vi "Auto.vi"() -> ()   [LabVIEW 2017]
uses:
  Control/Saurabh/prosucer_consumer_enum.ctl
  <vilib>/addons/database/NI_Database_API.lvlib
  Global/Global 1.vi
  <vilib>/Utility/file.llb/Read Delimited Spreadsheet (string).vi
  Global/DATA LOG.vi
  <vilib>/Utility/error.llb/DialogType.ctl
  <userlib>/_OpenG.lib/comparison/comparison.llb/String Changed__ogtk.vi
  <vilib>/addons/database/Connection.llb/DB Tools Open Connec (String).vi
panel:
  out "LOG DATA":string
  out "scanner value":string
  out "PRIVIOUS DATA":string
  out "array w/ subset deleted":dbl[](array[numeric])
  out "LOG DATA 2":dbl[](array[numeric])
  out "DATA":bool
  out "Boolean 6":bool
  out "Input 3":string
  out "resulting string":string
  out "error out 5":errorcluster
  out "BARCODE RECIPE 2":string(combo)
  out "match substring":string
  out "SHIFT_DATA":string[](array[string])
  out "length 2":i32
  out "length":i32
  out "Boolean 5":bool
  out "OP40 BARCODE STRING EMPRTY":bool
  out "OP30 BARCODE STRING EMPRTY":bool
  out "trimmed string":string
  out "Array":string[][](array[string])
  out "error out 3":errorcluster
  out "OP 61":T1 {"Cycle Time" format="%#.2g"; "Actual Flow (Lpm)" format="%#.2g"; "Pressure (Bar)" format="%#.2g"; "lt Pressure (Bar)" format="%#.2g"; "Actual Flow (ccm)" format="%#.2g"}
  out "error out":errorcluster
  out "OP 10 & OP 21":T2 {"SPRING AND SEAL PRESS CHECK LOAD(N)" format="%#.2g"; "CYCLE TIME" format="%#.2g"; "SPRING AND SEAL PRESS LOAD(N)" format="%#.2g"; "SPRING LOAD AT 13.4 mm(N)" format="%#.2g"; "SPRING LOAD AT 14 mm((N)" format="%#.2g"; "SPRING HEIGHT(mm)" format="%#.2g"; "SEAL PRESS LOAD(N)" format="%#.2g"}
  out "PLC COM.":bool
  out "STATION-4 2":T3 {"PARAMETER 10" format="%#.2g"; "PARAMETER 6" format="%#.2g"; "PARAMETER 7" format="%#.2g"; "PARAMETER 9" format="%#.2g"; "PARAMETER 8" format="%#.2g"; "CYCLE TIME" format="%#.2g"; "PARAMETER 5" format="%#.2g"; "PARAMETER 1" format="%#.2g"; "PARAMETER 2" format="%#.2g"; "PARAMETER 4" format="%#.2g"; "PARAMETER 3" format="%#.2g"}
  out "STATION-3 2":T3 {"PARAMETER 10" format="%#.2g"; "PARAMETER 6" format="%#.2g"; "PARAMETER 7" format="%#.2g"; "PARAMETER 9" format="%#.2g"; "PARAMETER 8" format="%#.2g"; "CYCLE TIME" format="%#.2g"; "PARAMETER 5" format="%#.2g"; "PARAMETER 1" format="%#.2g"; "PARAMETER 2" format="%#.2g"; "PARAMETER 4" format="%#.2g"; "PARAMETER 3" format="%#.2g"}
  out "STATION-2 2":T3 {"PARAMETER 10" format="%#.2g"; "PARAMETER 6" format="%#.2g"; "PARAMETER 7" format="%#.2g"; "PARAMETER 9" format="%#.2g"; "PARAMETER 8" format="%#.2g"; "CYCLE TIME" format="%#.2g"; "PARAMETER 5" format="%#.2g"; "PARAMETER 1" format="%#.2g"; "PARAMETER 2" format="%#.2g"; "PARAMETER 4" format="%#.2g"; "PARAMETER 3" format="%#.2g"}
  out "STATION-1 2":T4 {"PARAMETER 10" format="%#.2g"; "PARAMETER 6" format="%#.2g"; "PARAMETER 7" format="%#.2g"; "PARAMETER 9" format="%#.2g"; "PARAMETR 8" format="%#.2g"; "CYCLE TIME" format="%#.2g"; "PARAMETER 5" format="%#.2g"; "PARAMETER 1" format="%#.2g"; "PARAMETER 2" format="%#.2g"; "PARAMETER 4" format="%#.2g"; "PARAMETER 3" format="%#.2g"}
  out "stop":bool
  out "error out 2":errorcluster
  out "Shift 4":i32
  out "Time Stamp Out":timestamp[](array[timestamp]) format="%<%X>T"
  out "Time Stamp Out 4":timestamp[](array[timestamp]) format="%<%X>T"
  out "Shift_change":bool
  out "appended array":string[][](array[string])
  out "SHIFT_DATA 2":string[](array[string])
  out "SHIFT":string
  in  "error in (no error)":errorcluster
  in  "Tab Control":enum32{"Page 1", "Page 2"}(tab)
  out "OP - 20":T5
  out "Boolean 7":bool
  in  "NEXT":bool
  in  "stop 2":bool
  out "Boolean":bool
  out "Boolean 2":bool
  out "Boolean 3":bool
  out "Boolean 4":bool
  out "OP 40":T6 {"Calibration Pressure (Bar)" format="%#.2g"; "Fixing Ring Displacement (mm)" format="%#.2g"; "Cycle Time" format="%#.2g"; "Calibration Flow Rate (Lph)" format="%#.2g"; "Flushing Flow (Lph)" format="%#.2g"; "Flushing Pressure (Bar)" format="%#.2g"; "Calibration Displacement (mm)" format="%#.2g"; "Calibration Load (KgF)" format="%#.2g"}
  out "OP 60":T7 {"Cycle Time" format="%#.2g"; "Actual Flow (Lpm)" format="%#.2g"; "Pressure (Bar)" format="%#.2g"; "Pressure (Bar)" format="%#.2g"; "Actual Flow (ccm)" format="%#.2g"}
  out "OP - 10":T8
  out "OP - 30":T9
  in  "Add Button":bool
  in  "BARCODE RECIPE":string(combo)
  in  "Back":bool
  # "STATION 2 VALVE OPENING TEST"
  # "STATION 3 LEAK TEST"
  # "STATION 1 SPRING CHECKING"
  # "STATION 2 SPRING & SEAL ASSEMBLY"
  # "STATION 3 COVER & SUB ASSEMBLY"
  # "OP - 20"
  # "STATION 2 VALVE OPENING TEST"
  # "STATION 3 LEAK TEST"
  # "OP - 10"
  # "OP - 30"
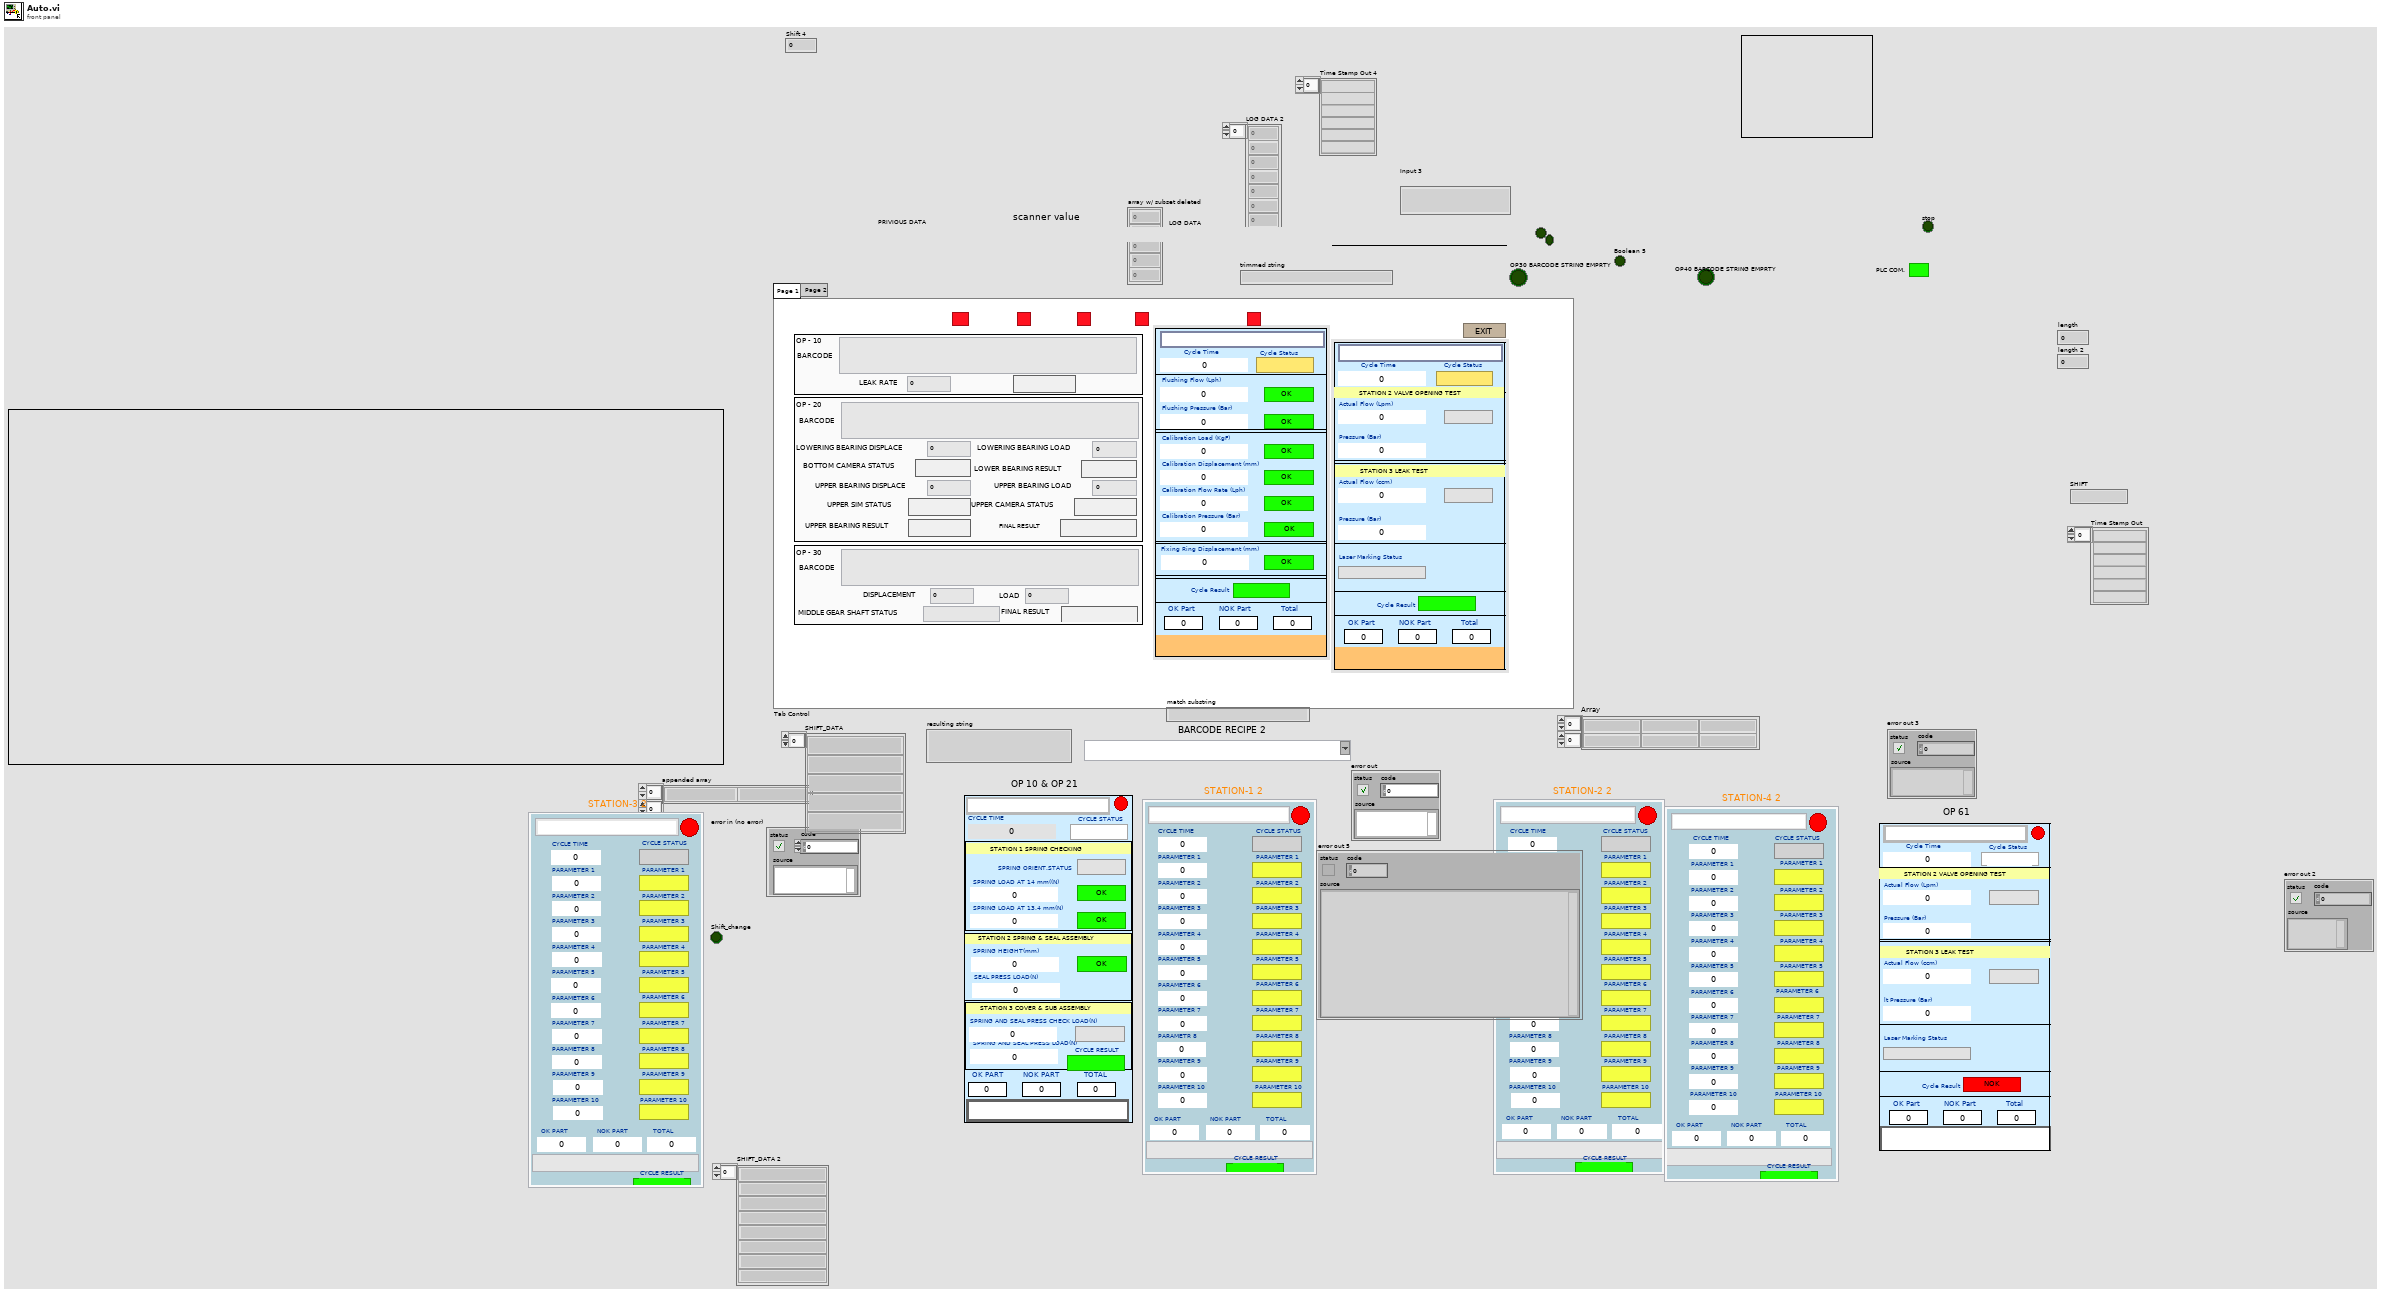
[diagram p1: front panel]
types:
  T1 = cluster{"BARCODE":string, "Cycle Time ":dbl, "Actual Flow (Lpm)":dbl, "Pressure (Bar)":dbl, "Actual Flow (ccm)":dbl, "lt Pressure (Bar)":dbl, "PARAMETER 5":dbl, "PARAMETER 6":dbl, "PARAMETER 7":dbl, "PARAMETER 8":dbl, "PARAMETER 9":dbl, "PARAMETER 10":dbl, "STATUS":string, "SCANNER":bool, "Cycle Status":bool, "VALVE OPENING TEST ACTUAL FLOW":bool, "LEAK TEST ACTUAL FLOW":bool, "Laser Marking Status":bool, "PARAMETER 4":bool, "PARAMETER 5":bool, "PARAMETER 6":bool, "PARAMETER 7":bool, "PARAMETER 8":bool, "PARAMETER 9":bool, "PARAMETER 10":bool, "OK Part":dbl, "NOK Part":dbl, "Total ":dbl, "Cycle Result":bool}
  T2 = cluster{"BARCODE":string, "CYCLE TIME":dbl, "SPRING LOAD AT 13.4 mm(N)":dbl, "SPRING LOAD AT 14 mm((N)":dbl, "SEAL PRESS LOAD(N)":dbl, "SPRING HEIGHT(mm)":dbl, "SPRING AND SEAL PRESS LOAD(N)":dbl, "SPRING AND SEAL PRESS CHECK LOAD(N)":dbl, "PARAMETER 7":dbl, "PARAMETR 8":dbl, "PARAMETER 9":dbl, "PARAMETER 10":dbl, "STATUS":string, "SCANNER":bool, "CYCLE STATUS":bool, "SPRING ORIENT.STATUS":bool, "SPRING LOAD AT 13.4 mm":bool, "SPRING LOAD AT 14 mm":bool, "SEAL PRESS LOAD(N)":bool, "SPRING HEIGHT(mm)":bool, "SPRING AND SEAL PRESS LOAD(N)":bool, "SPRING AND SEAL PRESS CHECK LOAD(N)":bool, "PARAMETER 8":bool, "PARAMETER 9":bool, "PARAMETER 10":bool, "OK PART":dbl, "NOK PART":dbl, "TOTAL ":dbl, "CYCLE RESULT":bool}
  T3 = cluster{"BARCODE":string, "CYCLE TIME":dbl, "PARAMETER 1":dbl, "PARAMETER 2":dbl, "PARAMETER 3":dbl, "PARAMETER 4":dbl, "PARAMETER 5":dbl, "PARAMETER 6":dbl, "PARAMETER 7":dbl, "PARAMETER 8":dbl, "PARAMETER 9":dbl, "PARAMETER 10":dbl, "STATUS":string, "SCANNER":bool, "CYCLE STATUS":bool, "PARAMETER 1":bool, "PARAMETER 2":bool, "PARAMETER 3":bool, "PARAMETER 4":bool, "PARAMETER 5":bool, "PARAMETER 6":bool, "PARAMETER 7":bool, "PARAMETER 8":bool, "PARAMETER 9":bool, "PARAMETER 10":bool, "OK PART":dbl, "NOK PART":dbl, "TOTAL ":dbl, "CYCLE RESULT":bool}
  T4 = cluster{"BARCODE":string, "CYCLE TIME":dbl, "PARAMETER 1":dbl, "PARAMETER 2":dbl, "PARAMETER 3":dbl, "PARAMETER 4":dbl, "PARAMETER 5":dbl, "PARAMETER 6":dbl, "PARAMETER 7":dbl, "PARAMETR 8":dbl, "PARAMETER 9":dbl, "PARAMETER 10":dbl, "STATUS":string, "SCANNER":bool, "CYCLE STATUS":bool, "PARAMETER 1":bool, "PARAMETER 2":bool, "PARAMETER 3":bool, "PARAMETER 4":bool, "PARAMETER 5":bool, "PARAMETER 6":bool, "PARAMETER 7":bool, "PARAMETER 8":bool, "PARAMETER 9":bool, "PARAMETER 10":bool, "OK PART":dbl, "NOK PART":dbl, "TOTAL ":dbl, "CYCLE RESULT":bool}
  T5 = cluster{"BARCODE":string, "LOWERING BEARING DISPLACE":dbl, "LOWERING BEARING LOAD":dbl, "BOTTOM CAMERA STATUS":bool, "LOWER BEARING RESULT":bool, "UPPER BEARING DISPLACE":dbl, "UPPER BEARING LOAD ":dbl, "UPPER SIM STATUS":bool, "UPPER CAMERA STATUS":bool, "UPPER BEARING RESULT":bool, "FINAL RESULT":bool}
  T6 = cluster{"BARCODE":string, "Cycle Time":dbl, "Flushing Flow (Lph)":dbl, "Flushing Pressure (Bar)":dbl, "Calibration Load (KgF) ":dbl, "Calibration Displacement (mm) ":dbl, "Calibration Flow Rate (Lph)":dbl, "Calibration Pressure (Bar)":dbl, "Fixing Ring Displacement (mm)":dbl, "PARAMETER 8":dbl, "PARAMETER 9":dbl, "PARAMETER 10":dbl, "STATUS":string, "SCANNER":bool, "Cycle Status":bool, "FLUSHING FLOW RATE":bool, "FLUSHING PRESSURE":bool, "CALIBRATION LOAD VALUE":bool, "CALIBRATION DISPLACEMENT VALUE":bool, "CALIBRATION FLOW RATE":bool, "CALIBRATION PRESSURE":bool, "FIXING RING DISPLACEMENT":bool, "PARAMETER 8":bool, "PARAMETER 9":bool, "PARAMETER 10":bool, "OK Part":dbl, "NOK Part":dbl, "Total ":dbl, "Cycle Result":bool}
  T7 = cluster{"BARCODE":string, "Cycle Time ":dbl, "Actual Flow (Lpm)":dbl, "Pressure (Bar)":dbl, "Actual Flow (ccm)":dbl, "Pressure (Bar)":dbl, "PARAMETER 5":dbl, "PARAMETER 6":dbl, "PARAMETER 7":dbl, "PARAMETER 8":dbl, "PARAMETER 9":dbl, "PARAMETER 10":dbl, "STATUS":string, "SCANNER":bool, "Cycle Status":bool, "VALVE OPENING TEST ACTUAL FLOW":bool, "LEAK TEST ACTUAL FLOW":bool, "Laser Marking Status":bool, "PARAMETER 4":bool, "PARAMETER 5":bool, "PARAMETER 6":bool, "PARAMETER 7":bool, "PARAMETER 8":bool, "PARAMETER 9":bool, "PARAMETER 10":bool, "OK Part":dbl, "NOK Part":dbl, "Total ":dbl, "Cycle Result":bool}
  T8 = cluster{"BARCODE":string, "LEAK RATE":dbl, "RESULT":bool}
  T9 = cluster{"BARCODE":string, "DISPLACEMENT":dbl, "LOAD":dbl, "MIDDLE GEAR SHAFT STATUS":string, "FINAL RESULT":bool}
  T10 = cluster{"OP - 10":cluster{"BARCODE":string, "LEAK RATE":dbl, "RESULT":bool}}
  T11 = typedef "prosucer_consumer_enum.ctl" = enum16{"SCAN1", "SCAN2", "SCAN3", "SCAN4", "STOP", "DATALOG1", "DATALOG2", "DATALOG3", "DATALOG4", "-1", "CYCLE_START1", "CYCLE_START2", "CYCLE_START3", "CYCLE_START4", "BARCODE RECIPE", "EMERGENCY STOP"}
  T12 = enum32{"invalid app kind", "Development System", "Run Time System", "Student Edition", "Embedded LabVIEW", "Evaluation", "Custom"}
  T13 = typedef "NI_Database_API.lvlib/Conn ObjectReference.ctl" = refnum<k1>
  T14 = typedef "DialogType.ctl" = u16
  T15 = cluster{"trimmed string":string, "SHIFT":string, "date/time string":string, dbl[], bool[], string}
  T16 = cluster{"SHIFT":string, "date/time string":string, dbl[], bool[], "CYCLE RESULT":bool, string}
  T17 = cluster{"SHIFT":string, "date/time string":string, dbl[], bool[], string}
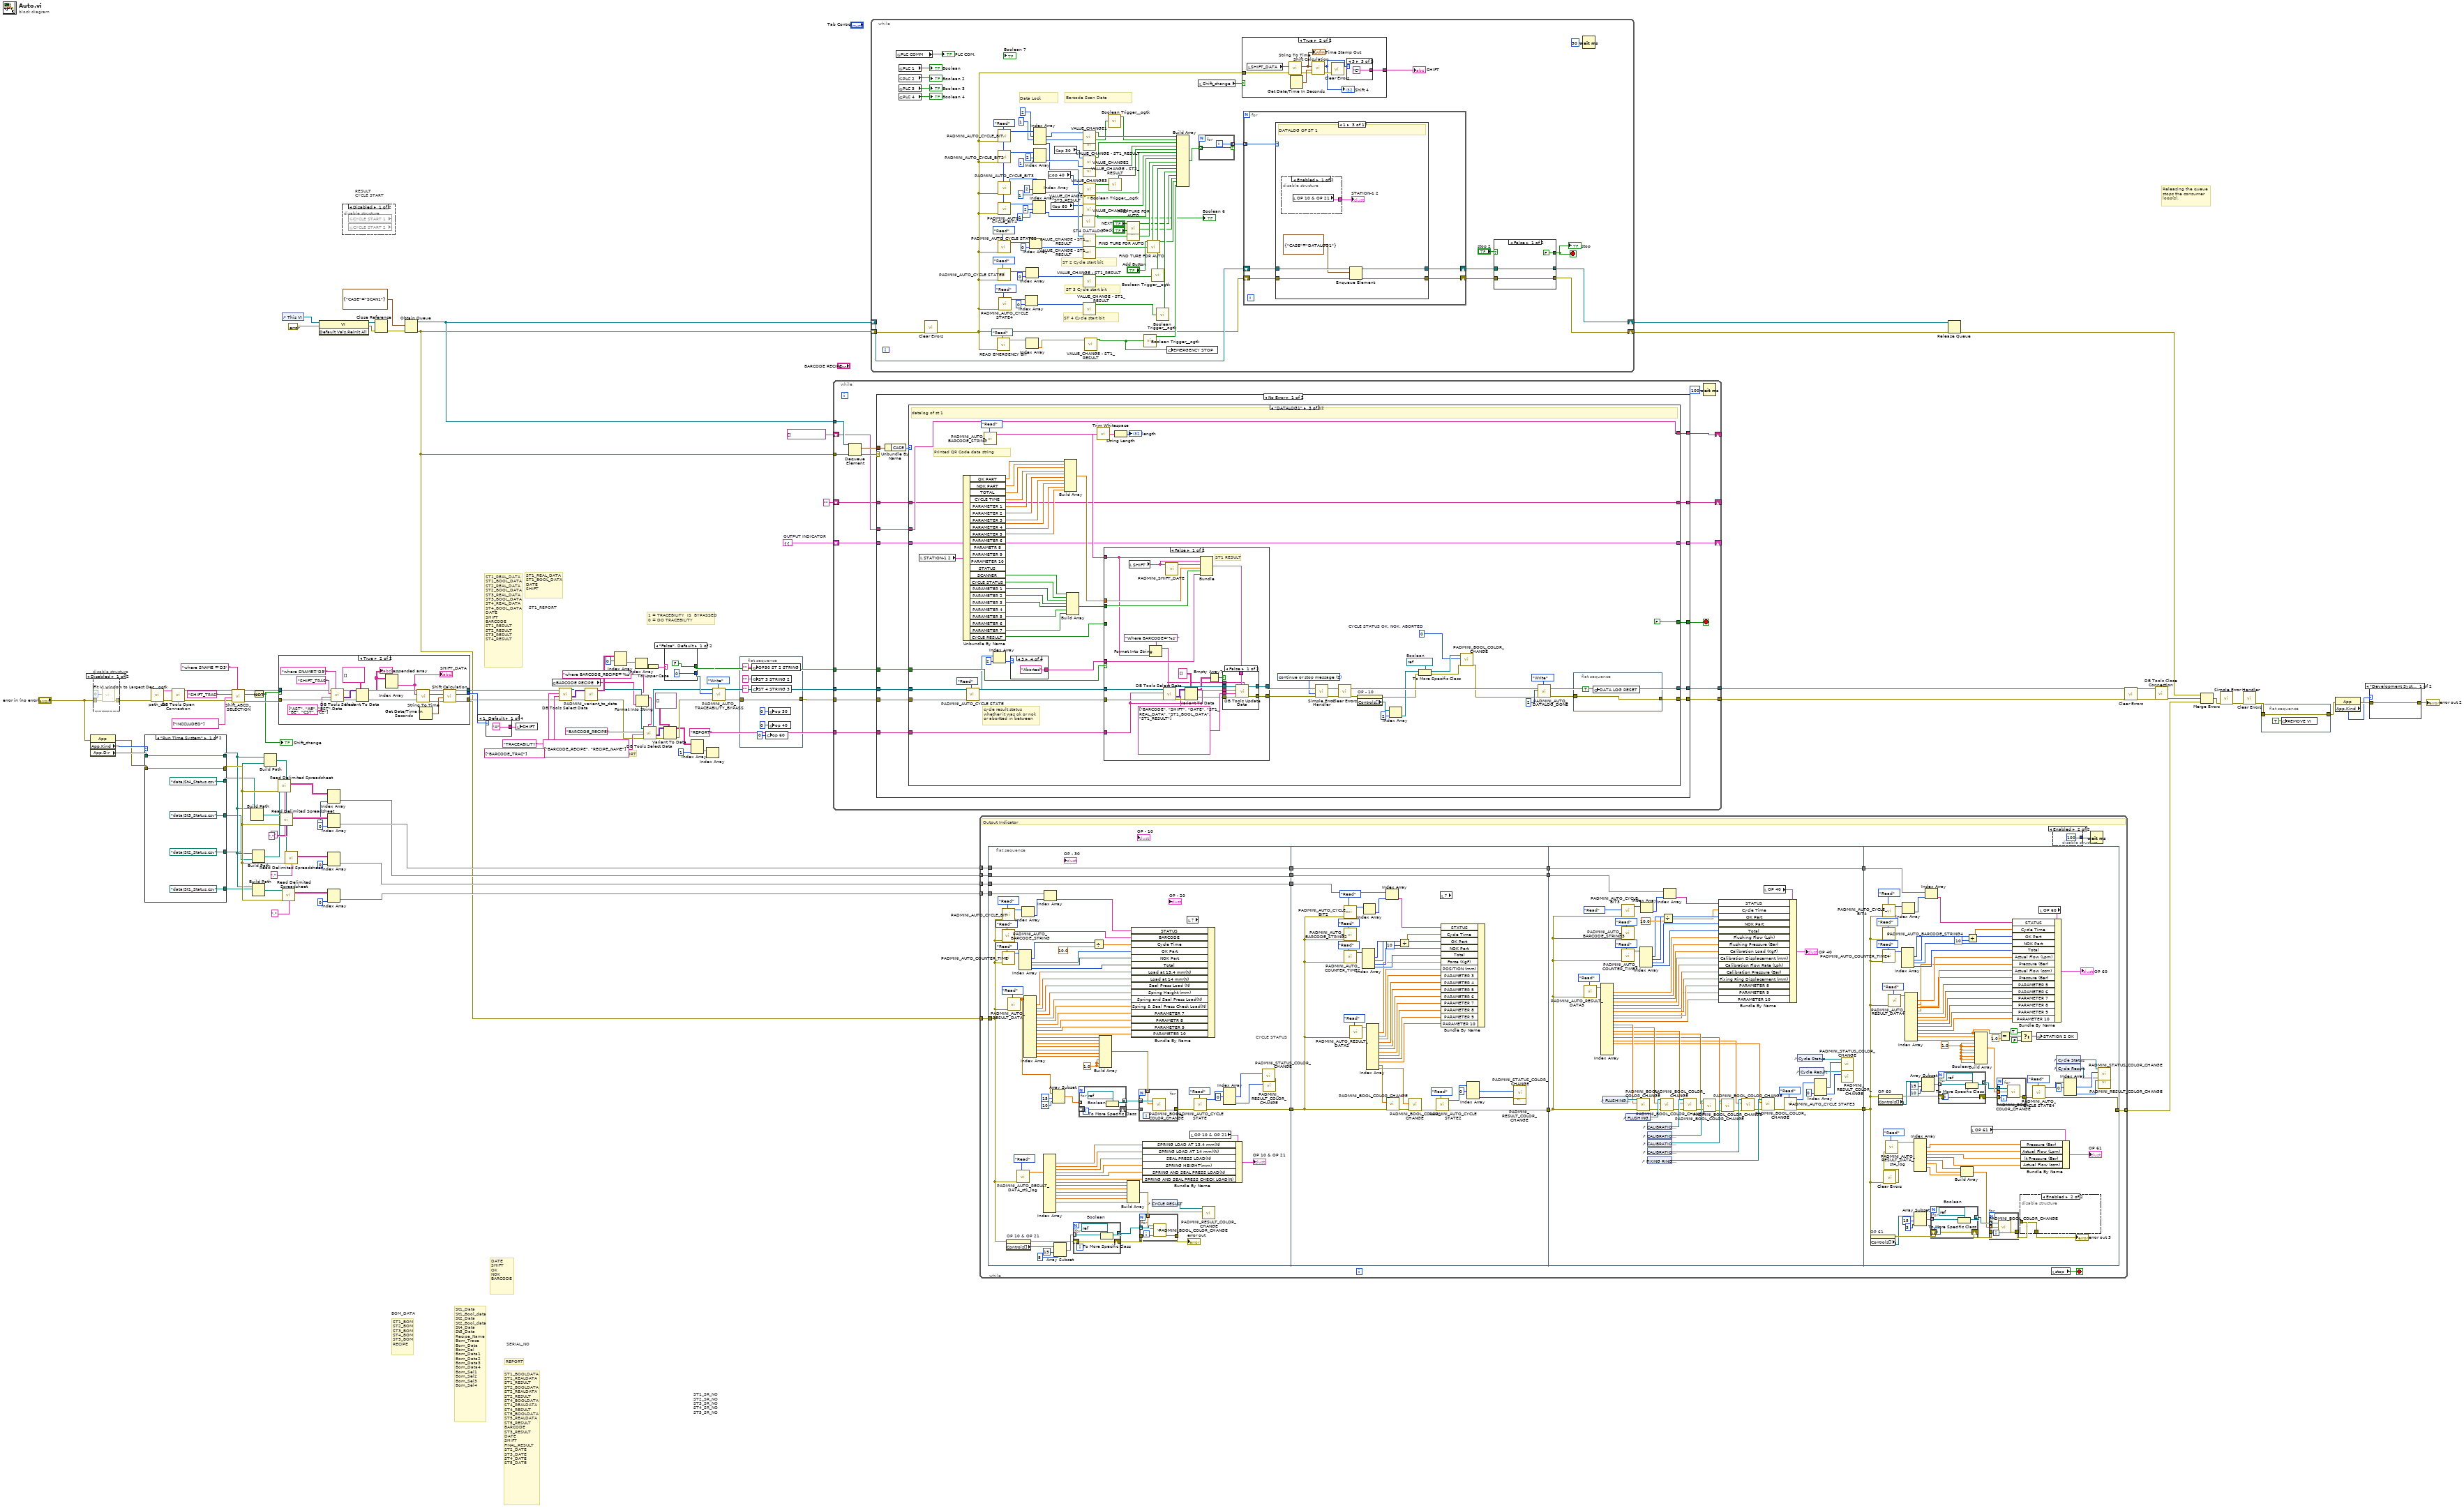
[diagram p0: block diagram]
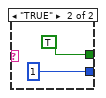
[diagram p3: hidden frame]
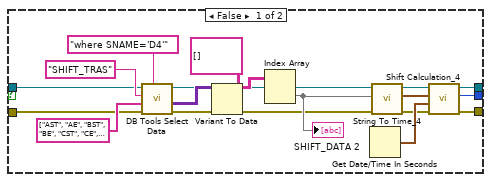
[diagram p4: hidden frame]
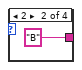
[diagram p5: hidden frame]
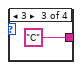
[diagram p6: hidden frame]
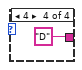
[diagram p7: hidden frame]
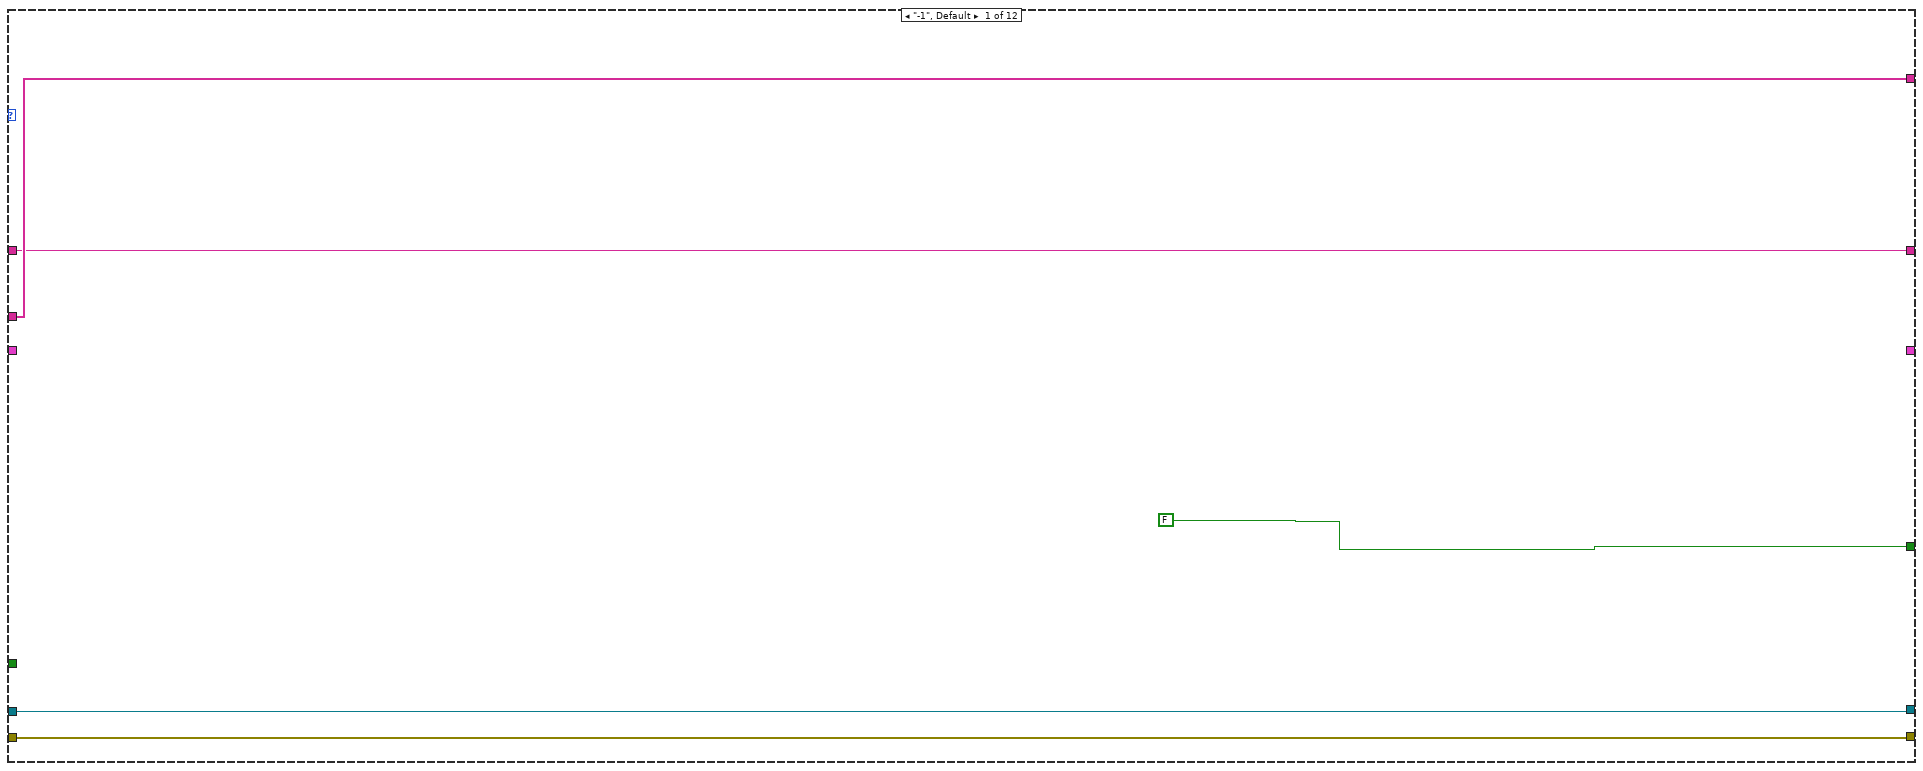
[diagram p9: hidden frame]
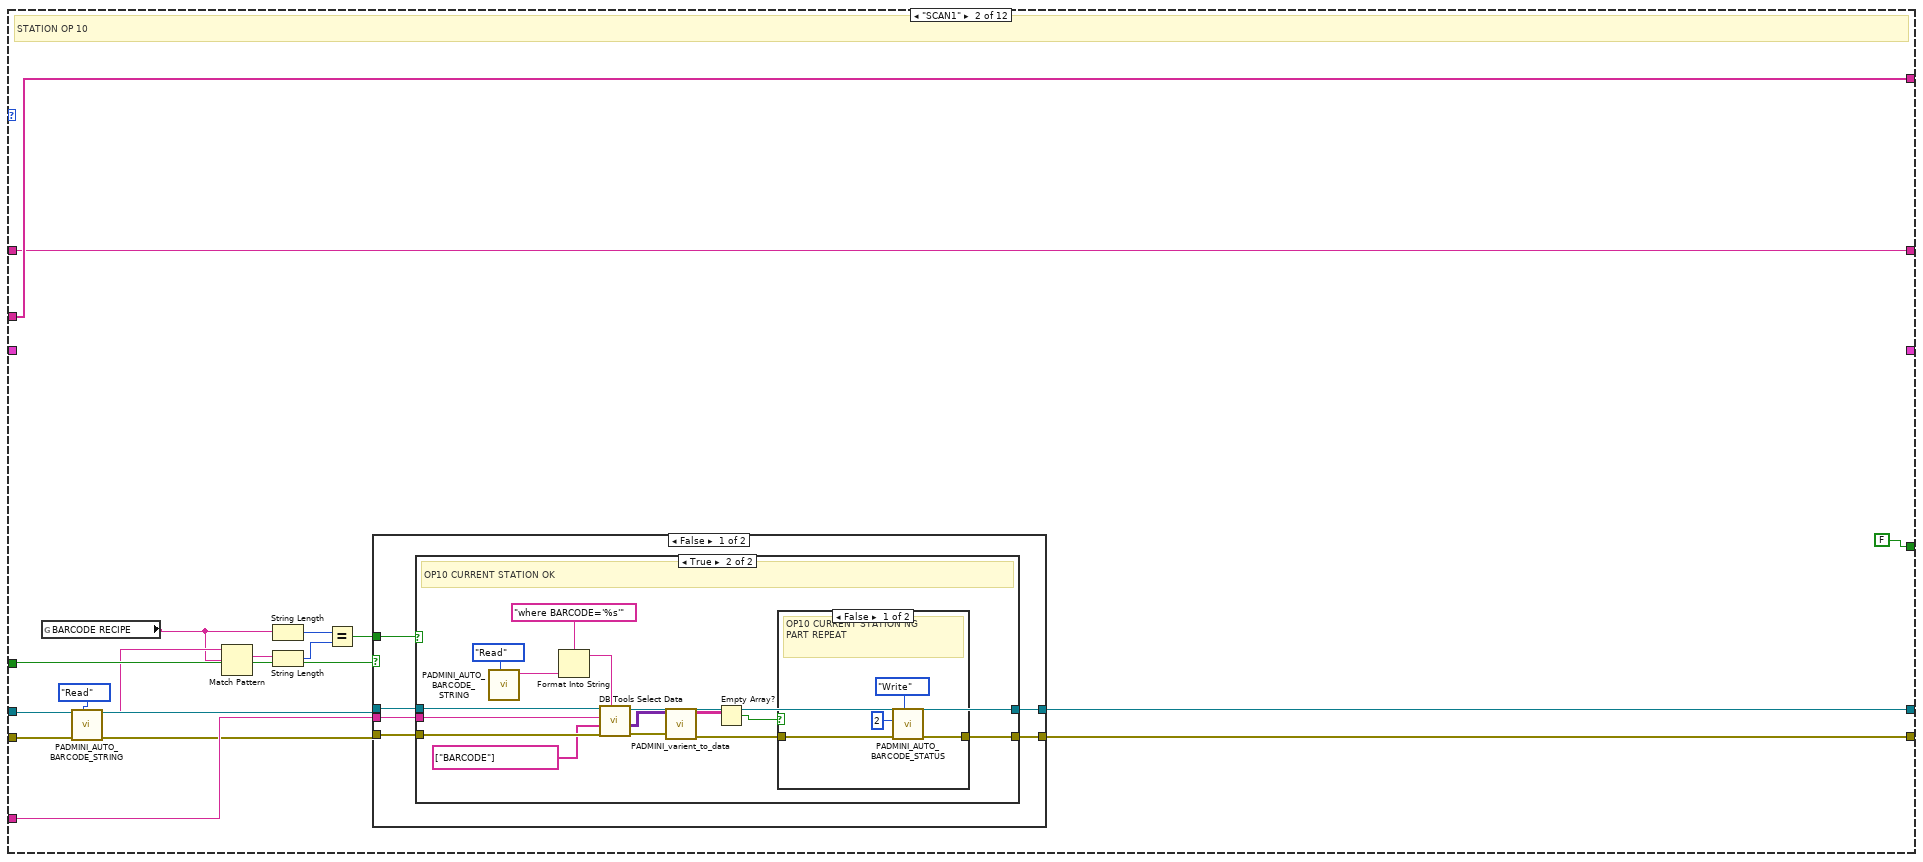
[diagram p10: hidden frame]
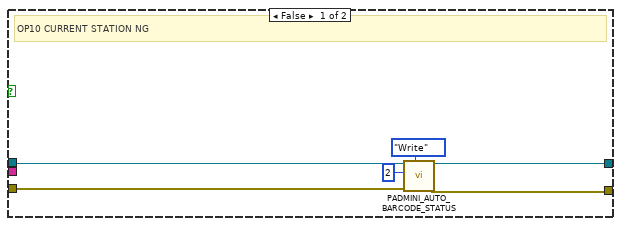
[diagram p11: hidden frame]
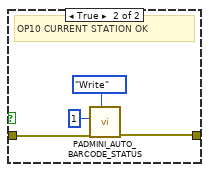
[diagram p12: hidden frame]
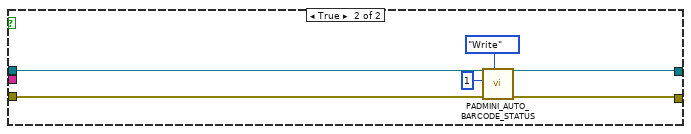
[diagram p13: hidden frame]
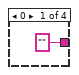
[diagram p14: hidden frame]
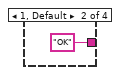
[diagram p15: hidden frame]
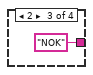
[diagram p16: hidden frame]
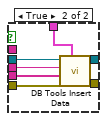
[diagram p17: hidden frame]
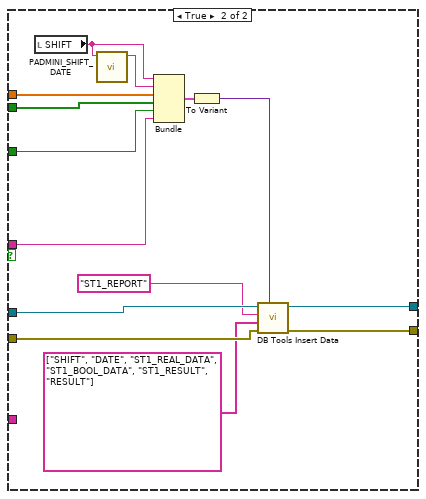
[diagram p18: hidden frame]
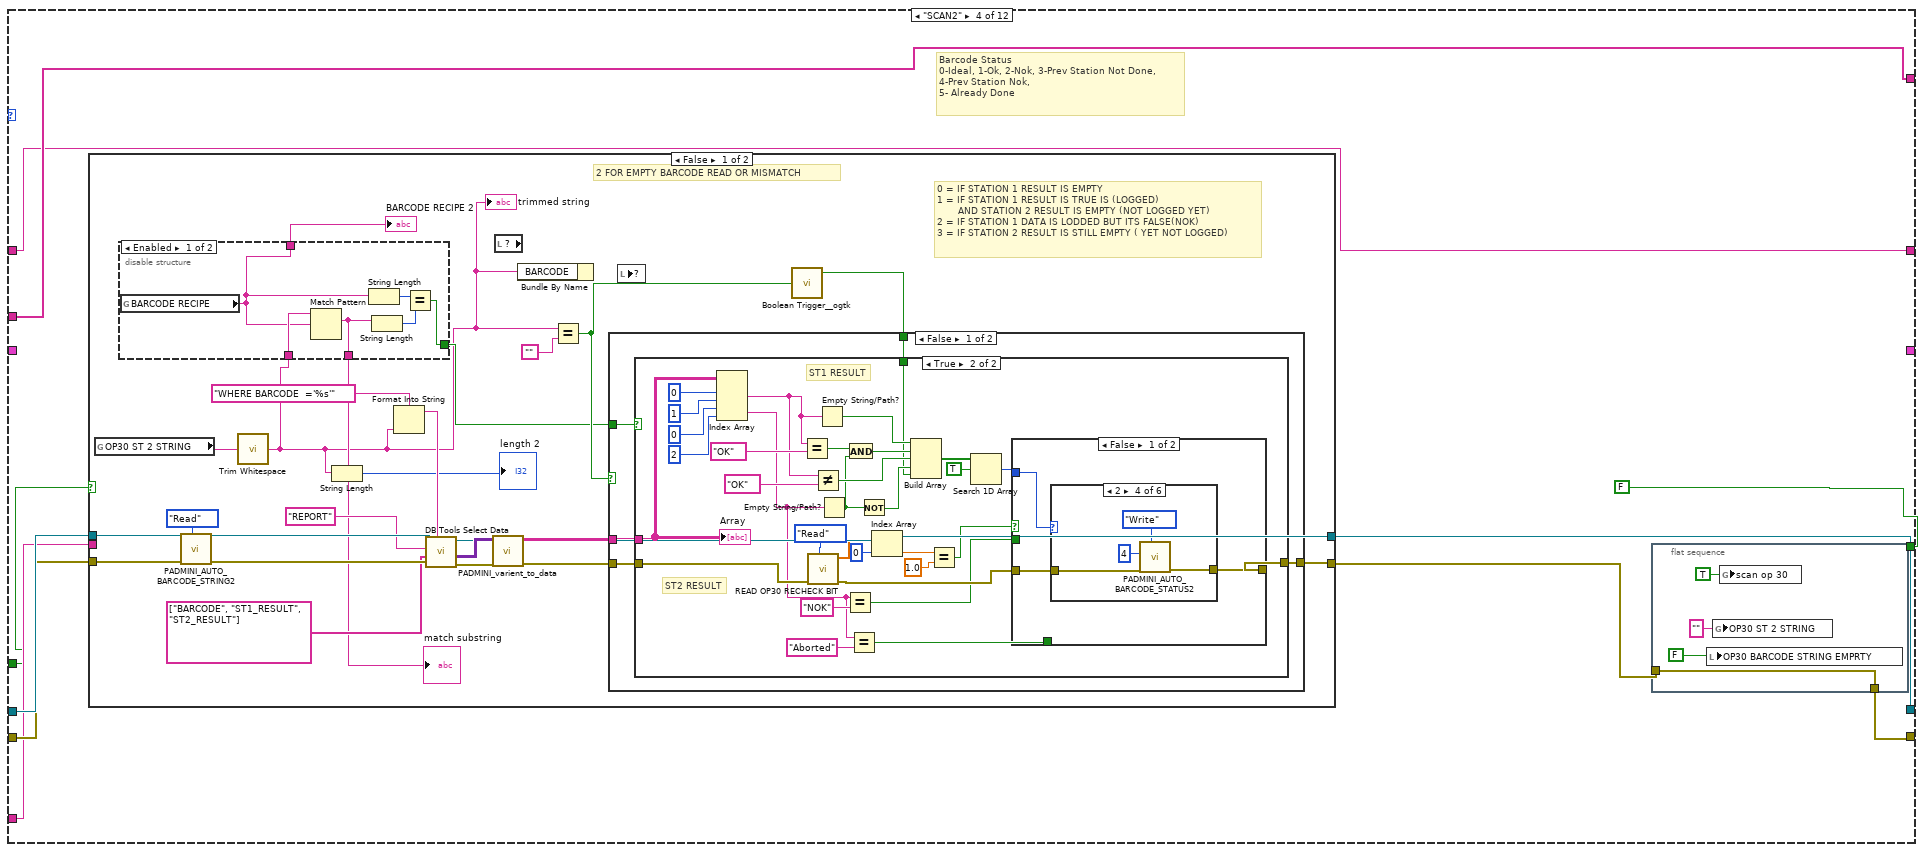
[diagram p19: hidden frame]
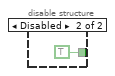
[diagram p20: hidden frame]
diagram:
  w1 = T10 {"OP - 10"={"BARCODE"="", "LEAK RATE"=0.0, "RESULT"=FALSE}}  # OUTPUT INDICATOR
  # "1 = TRACEBILITY  IS  BYPASSED\n0 = DO TRACEBILITY"
  # "ST1_REAL_DATA\nST1_BOOL_DATA\nST2_REAL_DATA\nST2_BOOL_DATA\nST3_REAL_DATA\nST3_BOOL_DATA\nST4_REAL_DATA\nST4_BOOL_DATA\nDATE\nSHIFT\nBARCODE\nST1_RESULT\nST2_RESULT\nST3_RESULT\nST4_RESULT"
  # "ST1_REPORT"
  # "ST1_REAL_DATA\nST1_BOOL_DATA\nDATE\nSHIFT"
  # "REPORT"
  # "DATE\nSHIFT\nOK\nNOK\nBARCODE"
  # "REPORT"
  # "ST1_BOOLDATA\nST1_REALDATA\nST1_RESULT\nST2_BOOLDATA\nST2_REALDATA\nST2_RESULT\nST4_BOOLDATA\nST4_REALDATA\nST4_RESULT\nST5_BOOLDATA\nST5_REALDATA\nST5_RESULT\nBARCODE\nST3_RESULT\nDATE\nSHIFT\nFINAL_RESULT\nST2_DATE\nST3_DATE\nST4_DATE\nST5_DATE"
  # "SERIAL_NO"
  # "ST1_SR_NO\nST2_SR_NO\nST3_SR_NO\nST4_SR_NO\nST5_SR_NO"
  # "RESULT\nCYCLE START"
  # "St1_Data\nSt1_Bool_data\nSt2_Data\nSt2_Bool_data\nSt4_Data\nSt5_Data\nRecipe_Name\nBom_Trace\nBom_Data\nBom_Sel\nBom_Data1\nBom_Data2\nBom_Data3\nBom_Data4\nBom_Sel1\nBom_Sel2\nBom_Sel3\nBom_Sel4"
  # "BOM_DATA"
  # "ST1_BOM\nST2_BOM\nST3_BOM\nST4_BOM\nST5_BOM\nRECIPE"
  # "Releasing the queue stops the consumer loop(s)."
  n1 = property class="App"(error in="error in (no error)") -> (error out=w84:errorcluster, "App.Kind"=w86:T12, "App.Dir"=w85:path)  [unwired: 1 in, 1 out]
  n2 = disable-structure shown="Disabled" {
    disable-tunnel: "error in (no error)" -> [w105 w106]
    disable-tunnel: [w104 w106] -> w37
    frame Disabled {
      n3 = call <userlib>:"Fit VI window to Largest Dec__ogtk.vi"("error in (no error)"=w105, "border spacing (2 px)"=0) -> ("error out"=w104:errorcluster)  [unwired: 4 in, 1 out]
    }
    frame Enabled {
    }
  }
  n4 = case shown="\"Run Time System\"" w86 {
    tunnel: w85 -> [w112 _]
    tunnel: [w112 w118] -> w49
    tunnel: w84 -> [w111 w117]
    tunnel: [w111 w117] -> w50
    tunnel: [path "data/St4_Status.csv" ("path") path "../data/St4_Status.csv" ("path")] -> w48
    tunnel: [path "data/St3_Status.csv" ("path") path "../data/St3_Status.csv" ("path")] -> w47
    tunnel: [path "data/St2_Status.csv" ("path") path "../data/St2_Status.csv" ("path")] -> w46
    tunnel: [path "data/St1_Status.csv" ("path") path "../data/St1_Status.csv" ("path")] -> w45
    frame "Run Time System" {
    }
    frame Default {
      n5 = Current VI's Path() -> (path=w119:path)
      n6 = Strip Path(path=w119) -> (stripped path=w118:path)  [unwired: 1 out]
    }
  }
  n7 = call "path_db.vi"("error in"=w37) -> ("error out"=w74:errorcluster, "resulting string"=w99:string)  [unwired: 9 in]
  n8 = call-poly <vilib>:"DB Tools Open Connection.vi"("error in (no error)"=w74, "connection information"=w99) -> ("error out"=w73:errorcluster, "connection reference"=w43:T13)  [unwired: 6 in]
  n9 = call "Shift_ABCD_SELECTION.vi"("Where"="where SNAME ='D3' ", "error in (no error)"=w73, "Array"=string[] ["INCCLUDED"], "table"="SHIFT_TRAS", "Refnum in"=w43) -> ("error out"=w90:errorcluster, "Boolean"=w89:bool, "Refnum out"=w91:T13)  [unwired: 4 in]
  n10 = Build Path(base path=w49, name or relative path=w48) -> (appended path=w64:path)
  n11 = Build Path(base path=w49, name or relative path=w47) -> (appended path=w61:path)
  n12 = Build Path(base path=w49, name or relative path=w45) -> (appended path=w53:path)
  n13 = Not(x=w89) -> (.not. x?=w88:bool)
  "Shift_change" <- w88
  n14 = Build Path(base path=w49, name or relative path=w46) -> (appended path=w56:path)
  n15 = call-poly <vilib>:"Read Delimited Spreadsheet.vi"("file path (dialog if empty)"=w61, "error in (no error)"=w50, "delimiter (\\t)"="," ("delimiter (\\t)")) -> ("all rows"=w60:string[][])  [unwired: 7 in, 5 out]
  n16 = case shown="True" w88 {
    tunnel: [w121 w145] -> w95
    tunnel: w91 -> [w124 w143]
    tunnel: w90 -> [w123 w142]
    tunnel: [w122 w141] -> w27
    tunnel: [w120 w135] -> w26
    frame False {
      n17 = call <vilib>:"DB Tools Select Data.vi"("condition"="where SNAME='D4'", "error in (no error)"=w123, "columns"=string[] ["AST", "AE", "BST", "BE", "CST", "CE", "DST", "DE"], "table"="SHIFT_TRAS", "connection reference"=w124) -> ("error out"=w130:errorcluster, "data"=w134:variant[][], "connection reference out"=w122:T13)  [unwired: 1 in]
      n18 = Variant To Data(error in=w130, type=string[][] [], Variant=w134) -> (data=w127:string[][], error out=w120:errorcluster)
      n19 = Index Array(array=w127) -> (element=w126:string[])  [unwired: 2 in]
      "SHIFT_DATA 2" <- w126
      n20 = Get Date/Time In Seconds() -> (seconds since 1Jan1904=w129:timestamp)
      n21 = call "String To Time_4.vi"("String Array In"=w126) -> ("Time Stamp Out"=w125:timestamp[])  [unwired: 9 in, 1 out]
      n22 = call "Shift Calculation_4.vi"("Current Time"=w129, "Time Stamp Out"=w125) -> ("Shift"=w121:i32)  [unwired: 8 in, 1 out]
    }
    frame True {
      n23 = call <vilib>:"DB Tools Select Data.vi"("condition"="where SNAME='D3'", "error in (no error)"=w142, "columns"=string[] ["AST", "AE", "BST", "BE", "CST", "CE"], "table"="SHIFT_TRAS", "connection reference"=w143) -> ("error out"=w147:errorcluster, "data"=w151:variant[][], "connection reference out"=w141:T13)  [unwired: 1 in]
      n24 = Variant To Data(error in=w147, type=string[][] [], Variant=w151) -> (data=w139:string[][], error out=w137:errorcluster)
      "appended array" <- w139
      n25 = Index Array(array=w139) -> (element=w138:string[])  [unwired: 2 in]
      "SHIFT_DATA" <- w138
      n26 = call "String To Time.vi"("error in (no error)"=w137, "String Array In"=w138) -> ("error out"=w136:errorcluster, "Time Stamp Out"=w144:timestamp[])  [unwired: 8 in]
      n27 = Get Date/Time In Seconds() -> (seconds since 1Jan1904=w146:timestamp)
      n28 = call "Shift Calculation.vi"("error in (no error)"=w136, "Current Time"=w146, "Time Stamp Out"=w144) -> ("error out"=w135:errorcluster, "Shift"=w145:i32)  [unwired: 7 in]
    }
  }
  n29 = call-poly <vilib>:"Read Delimited Spreadsheet.vi"("file path (dialog if empty)"=w64, "error in (no error)"=w50, "delimiter (\\t)"="," ("delimiter (\\t)")) -> ("all rows"=w65:string[][])  [unwired: 7 in, 5 out]
  n30 = control-ref of="This VI"() -> (w71:refnum<vi>)
  n31 = call-poly <vilib>:"Read Delimited Spreadsheet.vi"("file path (dialog if empty)"=w53, "error in (no error)"=w50, "delimiter (\\t)"="," ("delimiter (\\t)")) -> ("all rows"=w52:string[][])  [unwired: 7 in, 5 out]
  n32 = call-poly <vilib>:"Read Delimited Spreadsheet.vi"("file path (dialog if empty)"=w56, "error in (no error)"=w50, "delimiter (\\t)"="," ("delimiter (\\t)")) -> ("all rows"=w57:string[][])  [unwired: 7 in, 5 out]
  n33 = invoke class="VI" method="Default Vals.Reinit All"(reference=w71, error in=errorcluster {"status"=FALSE, "code"=0, "source"=""} ("error in (no error)")) -> (reference out=w69:refnum<vi>, error out=w70:errorcluster)  [unwired: 1 in, 1 out]
  n34 = Index Array(array=w60, index (col)=0 ("disabled index (col)")) -> (element=w40:string[])  [unwired: 1 in]
  n35 = Index Array(array=w65, index (col)=0 ("disabled index (col)")) -> (element=w42:string[])  [unwired: 1 in]
  n36 = Index Array(array=w57, index (col)=0 ("disabled index (col)")) -> (element=w39:string[])  [unwired: 1 in]
  n37 = Index Array(array=w52, index (col)=0 ("disabled index (col)")) -> (element=w41:string[])  [unwired: 1 in]
  n38 = disable-structure shown="Disabled" {
    frame Disabled {
      n39 = global read "Global 1.vi" "CYCLE START 1"() -> ()  [unwired: 1 out]
      n40 = global read "Global 1.vi" "CYCLE START 2"() -> ()  [unwired: 1 out]
    }
    frame Enabled {
    }
  }
  n41 = Close Reference(reference=w69, error in (no error)=w70) -> (error out=w67:errorcluster)
  n42 = Obtain Queue(element data type=cluster{"CASE":T11} {"CASE"=enum."SCAN1"}, error in (no error)=w67) -> (queue out=w100:refnum<queue>, error out=w19:errorcluster)  [unwired: 3 in, 1 out]
  n43 = case shown="1, Default" w95 {
    tunnel: ["A" "B" "C" "D"] -> w87
    frame 1, Default {
    }
    frame 2 {
    }
    frame 3 {
    }
    frame 4 {
    }
  }
  n44 = local write "SHIFT"(w87) -> ()
  n45 = global read "Global 1.vi" "BARCODE RECIPE"() -> (w7:string)
  n46 = call <vilib>:"DB Tools Select Data.vi"("error in (no error)"=w26, "columns"=string[] ["BARCODE_TRAC"], "table"="TRACEABILITY", "connection reference"=w27) -> ("error out"=w36:errorcluster, "data"=w35:variant[][], "connection reference out"=w13:T13)  [unwired: 2 in]
  n47 = call "PADMINI_varient_to_data.vi"("error in (no error)"=w36, "data"=w35) -> ("error out"=w11:errorcluster, "Array"=w34:string[][])  [unwired: 8 in]
  n48 = Index Array(array=w34, index (row)=0 ("disabled index (col)")) -> (element=w33:string[])  [unwired: 1 in]
  n49 = Index Array(array=w33) -> (element=w29:string)  [unwired: 1 in]
  n50 = Format Into String(format string="where BARCODE_RECIPE='%s' ", w7) -> (resulting string=w5:string)  [unwired: 2 in, 1 out]
  n51 = call <vilib>:"DB Tools Select Data.vi"("condition"=w5, "error in (no error)"=w11, "columns"=string[] ["BARCODE_RECIPE", "RECIPE_NAME"], "table"="BARCODE_RECIPE", "connection reference"=w13) -> ("error out"=w15:errorcluster, "data"=w14:variant[][], "connection reference out"=w12:T13)  [unwired: 1 in]
  n52 = To Upper Case(1:w29) -> (0:w28:string)
  n53 = Variant To Data(error in=w15, type=string[][] [], Variant=w14) -> (data=w8:string[][], error out=w10:errorcluster)
  n54 = case shown="\"False\", Default" w28 {
    tunnel: [FALSE ("BARCODE TRACEABILITY") TRUE ("BARCODE TRACEABILITY")] -> w18
    tunnel: [0 1] -> w24
    frame "False", Default {
    }
    frame "TRUE" {
    }
  }
  n55 = Index Array(array=w8, index (col)=1 ("disabled index (col)")) -> (element=w3:string[])  [unwired: 1 in]
  n56 = Index Array(array=w3) -> ()  [unwired: 1 in, 1 out]
  n57 = call "PADMINI_AUTO_TRACEABILITY_BYPASS.vi"("Enum"=enum16{"Read", "Write"}."Write", "error in (no error)"=w10, "I/P"=w24) -> ("error out"=w22:errorcluster)  [unwired: 7 in, 1 out]
  n58 = flat-sequence {
    tunnel: w22 -> [w163]
    tunnel: [w163] -> w21
    frame #0 {
      n59 = global write "DATA LOG.vi" "OP30 ST 2 STRING"("" ("OP30 ST 2 STRING")) -> ()
      n60 = global write "DATA LOG.vi" "ST 3 STRING 2"("" ("ST 3 STRING 2")) -> ()
      n61 = global write "DATA LOG.vi" "ST 4 STRING 3"("" ("ST 4 STRING 3")) -> ()
      n62 = global write "DATA LOG.vi" "op 60"(0 ("op 30")) -> ()
      n63 = global write "DATA LOG.vi" "op 30"(0 ("op 30")) -> ()
      n64 = global write "DATA LOG.vi" "op 40"(0 ("op 30")) -> ()
    }
  }
  n65 = while {
    tunnel: w100 -> [w184]
    tunnel: w19 -> [w180]
    tunnel: w21 -> [w179]
    tunnel: w12 -> [w178]
    tunnel: [w177] -> w98
    tunnel: [w176] -> w97
    tunnel: w18 -> [w175]
    tunnel: "REPORT" -> [w174]
    shift-right: [w172] -> _
    shift-left: string[] [] -> [w173]
    shift-right: [w171] -> _
    shift-left: "" ("trimmed string") -> [w170]
    shift-right: [w167] -> _
    shift-left: w1 -> [w168]
    stop <- w181 stop-if-true
    n66 = Dequeue Element(queue=w184, error in (no error)=w180) -> (element=w182:cluster{"CASE":T11}, error out=w183:errorcluster)  [unwired: 1 in, 2 out]
    n67 = case shown="No Error" w183 {
      tunnel: w182 -> [w199 _]
      tunnel: [w195 TRUE] -> w181
      tunnel: w179 -> [w196 w1182]
      tunnel: w178 -> [w197 w1181]
      tunnel: [w193 w1182] -> w177
      tunnel: [w194 w1181] -> w176
      tunnel: w175 -> [w192 _]
      tunnel: w174 -> [w191 _]
      tunnel: w173 -> [w190 w1180]
      tunnel: [w189 w1180] -> w172
      tunnel: [w188 w1179] -> w171
      tunnel: w170 -> [w187 w1179]
      tunnel: w168 -> [w186 _]
      tunnel: [w185 _] -> w167
      frame No Error {
        n68 = Unbundle By Name(w199) -> ("CASE"=w198:T11)
        n69 = case shown="\"DATALOG1\"" w198 {
          tunnel: w197 -> [w203 w220 w300 w384 w528 w655 w858 w930 w1013 w1152 w1167 w1174]
          tunnel: w196 -> [w202 w215 w285 w383 w527 w654 w841 w915 w1024 w1151 w1166 w1176]
          tunnel: [FALSE FALSE FALSE FALSE FALSE FALSE FALSE FALSE FALSE FALSE FALSE TRUE] -> w195
          tunnel: [w203 w217 w295 w381 w525 w652 w852 w924 w1044 w1134 w1167 w1173] -> w194
          tunnel: [w202 w218 w291 w378 w522 w650 w848 w921 w1040 w1129 w1166 w1175] -> w193
          tunnel: w192 -> [_ w212 w299 w380 w524 w651 w857 w929 w1047 _ _ _]
          tunnel: w191 -> [_ w219 w298 w382 w526 w653 w856 w928 w1008 _ _ _]
          tunnel: w190 -> [w201 w216 w277 w376 w521 w648 w839 w911 w1032 w1140 w1164 w1177]
          tunnel: [w201 w216 w277 w376 w521 w647 w839 w911 w1029 w1140 w1164 w1177] -> w189
          tunnel: [w200 w211 w273 w375 w520 w646 w834 w906 w1018 w1127 w1163 w1168] -> w188
          tunnel: w187 -> [w200 w211 w273 w375 w520 w645 w834 w906 w1018 w1127 w1163 w1168]
          tunnel: w186 -> [_ _ w261 _ _ _ _ _ _ _ _ _]
          tunnel: [_ _ w261 _ _ _ _ _ _ _ _ _] -> w185
          frame "-1", Default {
          }
          frame "SCAN1" {
            # "STATION OP 10"
            n70 = global read "Global 1.vi" "BARCODE RECIPE"() -> (w205:string)
            n71 = call "PADMINI_AUTO_BARCODE_STRING.vi"("Enum"=enum16{"Read", "Write"}."Read", "error in (no error)"=w215) -> ("error out"=w214:errorcluster, "Input 2"=w206:string)  [unwired: 8 in]
            n72 = Match Pattern(string=w206, regular expression=w205) -> (match substring=w209:string)  [unwired: 1 in, 3 out]
            n73 = String Length(string=w205) -> (length=w208:i32)
            n74 = String Length(string=w209) -> (length=w207:i32)
            n75 = Equal?(x=w208, y=w207) -> (x = y?=w213:bool)
            n76 = case shown="False" w212 {
              tunnel: w220 -> [w227 w260]
              tunnel: w214 -> [w226 w257]
              tunnel: w219 -> [w225 _]
              tunnel: [w224 w256] -> w218
              tunnel: [w223 w260] -> w217
              tunnel: w213 -> [w222 _]
              frame False {
                n77 = case shown="True" w222 {
                  tunnel: w227 -> [w228 w247]
                  tunnel: w226 -> [w230 w246]
                  tunnel: w225 -> [_ w245]
                  tunnel: [w229 w234] -> w224
                  tunnel: [w228 w233] -> w223
                  frame False {
                    # "OP10 CURRENT STATION NG"
                    n78 = call "PADMINI_AUTO_BARCODE_STATUS.vi"("Enum"=enum16{"Read", "Write"}."Write", "error in (no error)"=w230, "I/P"=u16 2) -> ("error out"=w229:errorcluster)  [unwired: 7 in, 1 out]
                  }
                  frame True {
                    # "OP10 CURRENT STATION OK"
                    n79 = call "PADMINI_AUTO_BARCODE_STRING.vi"("Enum"=enum16{"Read", "Write"}."Read") -> ("Input 2"=w243:string)  [unwired: 9 in, 1 out]
                    n80 = Format Into String(format string="where BARCODE='%s'", w243) -> (resulting string=w240:string)  [unwired: 2 in, 1 out]
                    n81 = call <vilib>:"DB Tools Select Data.vi"("condition"=w240, "error in (no error)"=w246, "columns"=string[] ["BARCODE"], "table"=w245, "connection reference"=w247) -> ("error out"=w239:errorcluster, "data"=w238:variant[][], "connection reference out"=w233:T13)  [unwired: 1 in]
                    n82 = call "PADMINI_varient_to_data.vi"("error in (no error)"=w239, "data"=w238) -> ("error out"=w235:errorcluster, "Array"=w237:string[][])  [unwired: 8 in]
                    n83 = Empty Array?(array=w237) -> (empty?=w236:bool)
                    n84 = case shown="False" w236 {
                      tunnel: w235 -> [w251 w255]
                      tunnel: [w250 w252] -> w234
                      frame False {
                        # "OP10 CURRENT STATION NG\nPART REPEAT"
                        n85 = call "PADMINI_AUTO_BARCODE_STATUS.vi"("Enum"=enum16{"Read", "Write"}."Write", "error in (no error)"=w251, "I/P"=u16 2) -> ("error out"=w250:errorcluster)  [unwired: 7 in, 1 out]
                      }
                      frame True {
                        # "OP10 CURRENT STATION OK"
                        n86 = call "PADMINI_AUTO_BARCODE_STATUS.vi"("Enum"=enum16{"Read", "Write"}."Write", "error in (no error)"=w255, "I/P"=u16 1) -> ("error out"=w252:errorcluster)  [unwired: 7 in, 1 out]
                      }
                    }
                  }
                }
              }
              frame True {
                n87 = call "PADMINI_AUTO_BARCODE_STATUS.vi"("Enum"=enum16{"Read", "Write"}."Write", "error in (no error)"=w257, "I/P"=u16 1) -> ("error out"=w256:errorcluster)  [unwired: 7 in, 1 out]
              }
            }
          }
          frame "DATALOG1" {
            w262 = u16 0  # CYCLE STATUS OK, NOK, ABORTED
            w267 = refnum<vi> refnum  # Boolean
            w275 = T14 2 items=["no dialog", "OK message", "continue or stop message", "OK message + warnings", "continue/stop + warnings"] ("type of dialog (OK msg:1)")
            # "cycle result status\nwhether it was ok or nok\nor abortted in between"
            # "Printed QR Code data string"
            # "datalog of st 1"
            n88 = local read "STATION-1 2"() -> (w316:T4)
            n89 = Unbundle By Name(w316) -> ("OK PART"=w308:dbl, "NOK PART"=w307:dbl, "TOTAL"=w306:dbl, "CYCLE TIME"=w315:dbl, "PARAMETER 1"=w314:dbl, "PARAMETER 2"=w313:dbl, "PARAMETER 3"=w312:dbl, "PARAMETER 4"=w311:dbl, "PARAMETER 5"=w310:dbl, "PARAMETER 6"=w309:dbl, "SCANNER"=w305:bool, "CYCLE STATUS"=w304:bool, "PARAMETER 1"=w303:bool, "PARAMETER 2"=w302:bool, "PARAMETER 3"=w301:bool, "PARAMETER 5"=w290:bool, "PARAMETER 7"=w289:bool, "CYCLE RESULT"=w288:bool)  [unwired: 6 out]
            n90 = call "PADMINI_AUTO_CYCLE STATE.vi"("Enum"=enum16{"Read", "Write"}."Read", "error in (no error)"=w285) -> ("error out"=w284:errorcluster, "Input 2"=w282:u16[])  [unwired: 8 in]
            n91 = call "PADMINI_AUTO_BARCODE_STRING.vi"("Enum"=enum16{"Read", "Write"}."Read") -> ("Input 2"=w278:string)  [unwired: 9 in, 1 out]
            n92 = Index Array(array=w282, index=2) -> (element=w263:u16)
            n93 = case shown="3" w263 {
              tunnel: ["" "OK" "NOK" "Aborted"] -> w286
              frame 0 {
              }
              frame 1, Default {
              }
              frame 2 {
              }
              frame 3 {
              }
            }
            n94 = Build Array(w308, w307, w306, w315, w314, w313, w312, w311, w310, w309) -> (w297:dbl[])
            n95 = Build Array(w305, w304, w303, w302, w301, w290, w289) -> (w296:bool[])
            n96 = call <vilib>:"Trim Whitespace.vi"("string"=w278) -> ("trimmed string"=w279:string)  [unwired: 1 in]
            n97 = case shown="False" w299 {
              tunnel: w300 -> [w335 w374]
              tunnel: w284 -> [w337 w373]
              tunnel: [w345 w372] -> w295
              tunnel: [w344 w371] -> w276
              tunnel: w298 -> [w332 _]
              tunnel: w279 -> [w329 _]
              tunnel: w297 -> [w341 w367]
              tunnel: w296 -> [w340 w366]
              tunnel: w288 -> [_ w362]
              tunnel: w286 -> [w339 w361]
              frame False {
                w331 = string[] ["BARCODE", "SHIFT", "DATE", "ST1_REAL_DATA", "ST1_BOOL_DATA", "ST1_RESULT"]
                # "ST1 RESULT"
                n98 = local read "SHIFT"() -> (w343:string)
                n99 = Format Into String(format string="Where BARCODE='%s' ", w329) -> (resulting string=w324:string)  [unwired: 2 in, 1 out]
                n100 = call <vilib>:"DB Tools Select Data.vi"("condition"=w324, "error in (no error)"=w337, "columns"=w331, "table"=w332, "connection reference"=w335) -> ("error out"=w333:errorcluster, "data"=w336:variant[][], "connection reference out"=w334:T13)  [unwired: 1 in]
                n101 = call "PADMINI_SHIFT_DATE.vi"("SHIFT"=w343) -> ("date/time string"=w342:string)  [unwired: 10 in]
                n102 = Variant To Data(error in=w333, type=string[][] [], Variant=w336) -> (data=w327:string[][], error out=w325:errorcluster)
                n103 = Bundle("trimmed string"=w329, "SHIFT"=w343, "date/time string"=w342, w341, w340, w339) -> (w338:T15)  [unwired: 1 in]
                n104 = Empty Array?(array=w327) -> (empty?=w326:bool)
                n105 = case shown="False" w326 {
                  tunnel: w334 -> [w350 w360]
                  tunnel: w325 -> [w349 w359]
                  tunnel: [w353 w358] -> w345
                  tunnel: [w352 w357] -> w344
                  tunnel: w331 -> [w347 w356]
                  tunnel: w332 -> [w348 w355]
                  tunnel: w338 -> [w351 w354]
                  tunnel: w324 -> [w346 _]
                  frame False {
                    n106 = call <vilib>:"DB Tools Update Data.vi"("condition"=w346, "data"=w351, "error in (no error)"=w349, "columns"=w347, "table"=w348, "connection reference"=w350) -> ("error out"=w352:errorcluster, "connection reference out"=w353:T13)  [unwired: 4 in]
                  }
                  frame True {
                    n107 = call <vilib>:"DB Tools Insert Data.vi"("data"=w354, "error in (no error)"=w359, "columns"=w356, "table"=w355, "connection reference"=w360) -> ("error out"=w357:errorcluster, "connection reference out"=w358:T13)  [unwired: 5 in]
                  }
                }
              }
              frame True {
                n108 = local read "SHIFT"() -> (w369:string)
                n109 = call "PADMINI_SHIFT_DATE.vi"("SHIFT"=w369) -> ("date/time string"=w368:string)  [unwired: 10 in]
                n110 = Bundle("SHIFT"=w369, "date/time string"=w368, w367, w366, "CYCLE RESULT"=w362, w361) -> (w365:T16)  [unwired: 1 in]
                n111 = To Variant(anything=w365) -> (Variant=w364:variant)
                n112 = call <vilib>:"DB Tools Insert Data.vi"("data"=w364, "error in (no error)"=w373, "columns"=string[] ["SHIFT", "DATE", "ST1_REAL_DATA", "ST1_BOOL_DATA", "ST1_RESULT", "RESULT"], "table"="ST1_REPORT", "connection reference"=w374) -> ("error out"=w371:errorcluster, "connection reference out"=w372:T13)  [unwired: 5 in]
              }
            }
            n113 = String Length(string=w279) -> (length=→"length":i32)
            n114 = call <vilib>:"Simple Error Handler.vi"("type of dialog (OK msg:1)"=w275, "error in (no error)"=w276) -> ("error out"=w274:errorcluster)  [unwired: 3 in, 4 out]
            n115 = call <vilib>:"Clear Errors.vi"("error in (no error)"=w274) -> ("error out"=w272:errorcluster)  [unwired: 5 in, 1 out]
            n116 = property on="OP - 10" class="Clust"(error in=w272) -> (error out=w266:errorcluster, "Controls[]"=w270:refnum<vi>[])  [unwired: 1 in, 1 out]
            n117 = Index Array(array=w270, index=2) -> (element=w268:refnum<vi>)
            n118 = To More Specific Class(target class=w267, reference=w268, error in=w266) -> (specific class reference=w271:refnum<vi>, error out=w265:errorcluster)
            n119 = call "PADMINI_BOOL_COLOR_CHANGE.vi"("error in (no error)"=w265, "Numeric"=w262, "Boolean in"=w271) -> ("error out"=w264:errorcluster)  [unwired: 8 in]
            n120 = call "PADMINI_AUTO_DATALOG_DONE.vi"("Enum"=enum16{"Read", "Write"}."Write", "error in (no error)"=w264, "I/P"=u16 2) -> ("error out"=w292:errorcluster)  [unwired: 7 in, 1 out]
            n121 = flat-sequence {
              tunnel: [w322] -> w291
              tunnel: w292 -> [w322]
              frame #0 {
                n122 = global write "DATA LOG.vi" "DATA LOG RESET"(TRUE ("DATA LOG RESET")) -> ()
              }
            }
          }
          frame "SCAN2" {
            # "Barcode Status\n0-Ideal, 1-Ok, 2-Nok, 3-Prev Station Not Done,\n4-Prev Station Nok,\n5- Already Done"
            n123 = case shown="False" w380 {
              tunnel: w384 -> [w411 w519]
              tunnel: w383 -> [w403 w516]
              tunnel: w382 -> [_ _]
              tunnel: [w406 w515] -> w379
              tunnel: [w404 w519] -> w381
              frame False {
                # "2 FOR EMPTY BARCODE READ OR MISMATCH"
                # "0 = IF STATION 1 RESULT IS EMPTY\n1 = IF STATION 1 RESULT IS TRUE IS (LOGGED)\n       AND STATION 2 RESULT IS EMPTY (NOT LOGGED YET)\n2 = IF STATION 1 DATA IS LODDED BUT ITS FALSE(NOK)\n3 = IF STATION 2 RESULT IS STILL EMPTY ( YET NOT LOGGED)"
                n124 = global read "DATA LOG.vi" "OP30 ST 2 STRING"() -> (w390:string)
                n125 = call "PADMINI_AUTO_BARCODE_STRING2.vi"("Enum"=enum16{"Read", "Write"}."Read", "error in (no error)"=w403) -> ("error out"=w402:errorcluster)  [unwired: 8 in, 1 out]
                n126 = call <vilib>:"Trim Whitespace.vi"("string"=w390) -> ("trimmed string"=w389:string)  [unwired: 1 in]
                "trimmed string" <- w389
                n127 = disable-structure shown="Enabled" {
                  disable-tunnel: [w415 TRUE] -> w393
                  disable-tunnel: [w414 _] -> w392
                  disable-tunnel: [w412 _] -> w391
                  disable-tunnel: w389 -> [w413 _]
                  frame Enabled {
                    n128 = global read "Global 1.vi" "BARCODE RECIPE"() -> (w412:string)
                    n129 = Match Pattern(string=w413, regular expression=w412) -> (match substring=w414:string)  [unwired: 1 in, 3 out]
                    n130 = String Length(string=w412) -> (length=w417:i32)
                    n131 = String Length(string=w414) -> (length=w416:i32)
                    n132 = Equal?(x=w417, y=w416) -> (x = y?=w415:bool)
                  }
                  frame Disabled {
                  }
                }
                "match substring" <- w392
                "BARCODE RECIPE 2" <- w391
                n133 = String Length(string=w389) -> (length=→"length 2":i32)
                n134 = Format Into String(format string="WHERE BARCODE  ='%s'", w389) -> (resulting string=w398:string)  [unwired: 2 in, 1 out]
                n135 = call <vilib>:"DB Tools Select Data.vi"("condition"=w398, "error in (no error)"=w402, "columns"=string[] ["BARCODE", "ST1_RESULT", "ST2_RESULT"], "table"="REPORT", "connection reference"=w411) -> ("error out"=w409:errorcluster, "data"=w408:variant[][], "connection reference out"=w404:T13)  [unwired: 1 in]
                n136 = call "PADMINI_varient_to_data.vi"("error in (no error)"=w409, "data"=w408) -> ("error out"=w407:errorcluster, "Array"=w405:string[][])  [unwired: 8 in]
                n137 = local read item#-1() -> ()  [unwired: 1 out]
                n138 = Bundle By Name("BARCODE"=w389) -> ()  [unwired: 1 in, 1 out]
                n139 = Equal?(x=w389, y="") -> (x = y?=w395:bool)
                n140 = local read item#-1() -> ()  [unwired: 1 in]
                n141 = call <userlib>:"Boolean Trigger__ogtk.vi"("Boolean Input"=w395) -> ("Rising Edge"=w397:bool)  [unwired: 1 in, 1 out]
                n142 = case shown="False" w395 {
                  selector: w395 -> [_ w514]
                  tunnel: w407 -> [w423 w512]
                  tunnel: [w422 w511] -> w406
                  tunnel: w405 -> [w421 _]
                  tunnel: w397 -> [w420 _]
                  tunnel: w393 -> [w419 _]
                  frame False {
                    n143 = case shown="True" w419 {
                      tunnel: w423 -> [w425 w440]
                      tunnel: [w424 w459] -> w422
                      tunnel: w421 -> [_ w458]
                      tunnel: w420 -> [_ w430]
                      frame False {
                        n144 = call "PADMINI_AUTO_BARCODE_STATUS2.vi"("Enum"=enum16{"Read", "Write"}."Write", "error in (no error)"=w425, "I/P"=u16 2) -> ("error out"=w424:errorcluster)  [unwired: 7 in, 1 out]
                      }
                      frame True {
                        # "ST2 RESULT"
                        # "ST1 RESULT"
                        n145 = Index Array(array=w458, index (row) #1=0 ("index (row)"), index (col) #1=1 ("disabled index (col)"), index (row) #2=0 ("index (row)"), index (col) #2=2 ("disabled index (col)")) -> (element #1=w436:string, element #2=w432:string)
                        n146 = Equal?(x=w436, y="OK") -> (x = y?=w437:bool)
                        n147 = call "READ OP30 RECHECK BIT.vi"("Enum"=enum16{"Read", "Write"}."Read", "error in (no error)"=w440) -> ("error out"=w439:errorcluster, "Input 2"=w445:dbl[])  [unwired: 8 in]
                        n148 = Not Equal?(x=w436, y="OK") -> (x != y?=w454:bool)
                        n149 = Empty String/Path?(string/path=w436) -> (empty?=w455:bool)
                        n150 = Empty String/Path?(string/path=w432) -> (empty?=w447:bool)
                        n151 = Equal?(x=w432, y="NOK") -> (x = y?=w429:bool)
                        n152 = And(x=w437, y=w447) -> (x .and. y?=w448:bool)
                        n153 = Equal?(x=w432, y="Aborted") -> (x = y?=w428:bool)
                        n154 = Not(x=w447) -> (.not. x?=w434:bool)
                        n155 = Index Array(array=w445, index=0) -> (element=w444:dbl)
                        n156 = Build Array(w455, w448, w454, w434, w430) -> (w453:bool[])
                        n157 = Equal?(x=w444, y=1.0) -> (x = y?=w438:bool)
                        n158 = Search 1D Array(1D array=w453, element=TRUE) -> (index of element=w451:i32)  [unwired: 1 in]
                        n159 = case shown="False" w438 {
                          tunnel: [w462 w489] -> w459
                          tunnel: w451 -> [w461 _]
                          tunnel: w439 -> [w460 w490]
                          tunnel: w429 -> [_ w488]
                          tunnel: w428 -> [_ w487]
                          frame False {
                            n160 = case shown="2" w461 {
                              tunnel: w460 -> [w464 w468 w474 w478 w482 w486]
                              tunnel: [w463 w467 w471 w475 w479 w483] -> w462
                              frame -1, Default {
                                n161 = call "PADMINI_AUTO_BARCODE_STATUS2.vi"("Enum"=enum16{"Read", "Write"}."Write", "error in (no error)"=w464, "I/P"=u16 0) -> ("error out"=w463:errorcluster)  [unwired: 7 in, 1 out]
                              }
                              frame 0 {
                                n162 = call "PADMINI_AUTO_BARCODE_STATUS2.vi"("Enum"=enum16{"Read", "Write"}."Write", "error in (no error)"=w468, "I/P"=u16 3) -> ("error out"=w467:errorcluster)  [unwired: 7 in, 1 out]
                              }
                              frame 1 {
                                n163 = call "PADMINI_AUTO_BARCODE_STATUS2.vi"("Enum"=enum16{"Read", "Write"}."Write", "error in (no error)"=w474, "I/P"=u16 1) -> ("error out"=w471:errorcluster)  [unwired: 7 in, 1 out]
                              }
                              frame 2 {
                                n164 = call "PADMINI_AUTO_BARCODE_STATUS2.vi"("Enum"=enum16{"Read", "Write"}."Write", "error in (no error)"=w478, "I/P"=u16 4) -> ("error out"=w475:errorcluster)  [unwired: 7 in, 1 out]
                              }
                              frame 3 {
                                n165 = call "PADMINI_AUTO_BARCODE_STATUS2.vi"("Enum"=enum16{"Read", "Write"}."Write", "error in (no error)"=w482, "I/P"=u16 5) -> ("error out"=w479:errorcluster)  [unwired: 7 in, 1 out]
                              }
                              frame 4 {
                                n166 = call "PADMINI_AUTO_BARCODE_STATUS2.vi"("Enum"=enum16{"Read", "Write"}."Write", "error in (no error)"=w486, "I/P"=u16 2) -> ("error out"=w483:errorcluster)  [unwired: 7 in, 1 out]
                              }
                            }
                          }
                          frame True {
                            n167 = case shown="True" w488 {
                              tunnel: w490 -> [w493 w507]
                              tunnel: [w492 w506] -> w489
                              tunnel: w487 -> [w491 _]
                              frame False {
                                n168 = case shown="True" w491 {
                                tunnel: w493 -> [w500 w503]
                                tunnel: [w494 w502] -> w492
                                frame False {
                                n169 = global write "Global 1.vi" "RECHECK RESULT OK"(TRUE ("RECHECK RESULT OK")) -> ()
                                n170 = call "RESET RECHECK OP40 BIT.vi"("Enum"=enum16{"Read", "Write"}."Write", "error in (no error)"=w500, "Array"=u16[] [0]) -> ("error out"=w495:errorcluster)  [unwired: 7 in, 1 out]
                                n171 = call "PADMINI_AUTO_BARCODE_STATUS2.vi"("Enum"=enum16{"Read", "Write"}."Write", "error in (no error)"=w495, "I/P"=u16 5) -> ("error out"=w494:errorcluster)  [unwired: 7 in, 1 out]
                                }
                                frame True {
                                n172 = call "PADMINI_AUTO_BARCODE_STATUS2.vi"("Enum"=enum16{"Read", "Write"}."Write", "error in (no error)"=w503, "I/P"=u16 1) -> ("error out"=w502:errorcluster)  [unwired: 7 in, 1 out]
                                }
                                }
                              }
                              frame True {
                                n173 = call "PADMINI_AUTO_BARCODE_STATUS2.vi"("Enum"=enum16{"Read", "Write"}."Write", "error in (no error)"=w507, "I/P"=u16 1) -> ("error out"=w506:errorcluster)  [unwired: 7 in, 1 out]
                              }
                            }
                          }
                        }
                        "Array" <- w458
                      }
                    }
                  }
                  frame True {
                    n174 = call "PADMINI_AUTO_BARCODE_STATUS2.vi"("Enum"=enum16{"Read", "Write"}."Write", "error in (no error)"=w512, "I/P"=u16 2) -> ("error out"=w511:errorcluster)  [unwired: 7 in, 1 out]
                    "OP30 BARCODE STRING EMPRTY" <- w514
                  }
                }
              }
              frame True {
                n175 = call "PADMINI_AUTO_BARCODE_STATUS2.vi"("Enum"=enum16{"Read", "Write"}."Write", "error in (no error)"=w516, "I/P"=u16 1) -> ("error out"=w515:errorcluster)  [unwired: 7 in, 1 out]
              }
            }
            n176 = flat-sequence {
              tunnel: [w388] -> w378
              tunnel: w379 -> [w388]
              frame #0 {
                n177 = local write "OP30 BARCODE STRING EMPRTY"(FALSE ("Boolean 5")) -> ()
                n178 = global write "DATA LOG.vi" "OP30 ST 2 STRING"("" ("OP30 ST 2 STRING")) -> ()
                n179 = global write "DATA LOG.vi" "scan op 30"(TRUE ("scan op 30")) -> ()
              }
            }
          }
          frame "SCAN3" {
            n180 = case shown="False" w524 {
              tunnel: w528 -> [w554 w644]
              tunnel: w527 -> [w553 w642]
              tunnel: w526 -> [w552 _]
              tunnel: [w543 w641] -> w523
              tunnel: [w546 w644] -> w525
              frame False {
                # "Barcode Status\n0-Ideal, 1-Ok, 2-Nok, 3-Prev Station Not Done,\n4-Prev Station Nok,\n5- Already Done"
                # "0 = IF STATION 1 RESULT IS EMPTY\n1 = IF STATION 1 RESULT IS TRUE IS (LOGGED)\n       AND STATION 2 RESULT IS EMPTY (NOT LOGGED YET)\n2 = IF STATION 1 DATA IS LODDED BUT ITS FALSE(NOK)\n3 = IF STATION 2 RESULT IS STILL EMPTY ( YET NOT LOGGED)"
                n181 = global read "DATA LOG.vi" "ST 3 STRING 2"() -> (w541:string)
                n182 = local read "OP 40"() -> (w538:T6)
                n183 = call <vilib>:"Trim Whitespace.vi"("string"=w541) -> ("trimmed string"=w536:string)  [unwired: 1 in]
                n184 = disable-structure shown="Enabled" {
                  disable-tunnel: w536 -> [w556 _]
                  disable-tunnel: [w557 TRUE] -> w535
                  frame Enabled {
                    (unwired) "False"
                    (unwired) "True"
                    n185 = global read "Global 1.vi" "BARCODE RECIPE"() -> (w555:string)
                    n186 = Match Pattern(string=w556, regular expression=w555) -> (match substring=w560:string)  [unwired: 1 in, 3 out]
                    n187 = String Length(string=w555) -> (length=w559:i32)
                    n188 = String Length(string=w560) -> (length=w558:i32)
                    n189 = Equal?(x=w559, y=w558) -> (x = y?=w557:bool)
                  }
                  frame Disabled {
                  }
                }
                n190 = Bundle By Name(cluster=w538, "BARCODE"=w536) -> (w537:T6)
                n191 = Format Into String(format string="where BARCODE='%s'", w536) -> (resulting string=w549:string)  [unwired: 2 in, 1 out]
                n192 = call <vilib>:"DB Tools Select Data.vi"("condition"=w549, "error in (no error)"=w553, "columns"=string[] ["BARCODE", "ST2_RESULT", "ST3_RESULT"], "table"=w552, "connection reference"=w554) -> ("error out"=w548:errorcluster, "data"=w547:variant[][], "connection reference out"=w546:T13)  [unwired: 1 in]
                n193 = Equal?(x=w536, y="") -> (x = y?=w539:bool)
                n194 = local write "OP 40"(w537) -> ()
                n195 = case shown="False" w539 {
                  selector: w539 -> [_ w639]
                  tunnel: w548 -> [w566 w637]
                  tunnel: w547 -> [w565 _]
                  tunnel: [w564 w637] -> w544
                  tunnel: [w563 2] -> w542
                  tunnel: w535 -> [w562 _]
                  frame False {
                    n196 = case shown="True" w562 {
                      tunnel: w566 -> [w567 w603]
                      tunnel: w565 -> [_ w602]
                      tunnel: [w567 w593] -> w564
                      tunnel: [u16 2 ("I/P") w592] -> w563
                      frame False {
                      }
                      frame True {
                        (unwired) "OK"
                        (unwired) "OK"
                        n197 = call "PADMINI_varient_to_data.vi"("error in (no error)"=w603, "data"=w602) -> ("error out"=w574:errorcluster, "Array"=w594:string[][])  [unwired: 8 in]
                        n198 = Index Array(array=w594, index (row) #1=0 ("index (row)"), index (col) #1=1 ("disabled index (col)"), index (row) #2=0 ("index (row)"), index (col) #2=2 ("disabled index (col)")) -> (element #1=w577:string, element #2=w571:string)
                        n199 = call <vilib>:"Clear Errors.vi"("error in (no error)"=w574) -> ("error out"=w573:errorcluster)  [unwired: 5 in, 1 out]
                        n200 = Not Equal?(x=w577, y="OK") -> (x != y?=w600:bool)
                        n201 = Equal?(x=w577, y="OK") -> (x = y?=w579:bool)
                        n202 = Empty String/Path?(string/path=w577) -> (empty?=w601:bool)
                        n203 = Empty String/Path?(string/path=w571) -> (empty?=w595:bool)
                        n204 = call "RECHECK READ BIT.vi"("Enum"=enum16{"Read", "Write"}."Read", "error in (no error)"=w573) -> ("error out"=w580:errorcluster, "Input 2"=w584:dbl[])  [unwired: 8 in]
                        n205 = Equal?(x=w571, y="Aborted") -> (x = y?=w569:bool)
                        n206 = Equal?(x=w571, y="NOK") -> (x = y?=w570:bool)
                        n207 = And(x=w579, y=w595) -> (x .and. y?=w596:bool)
                        n208 = Not(x=w595) -> (.not. x?=w591:bool)
                        n209 = Index Array(array=w584, index=0) -> (element=w585:dbl)
                        n210 = Build Array(w601, w596, w600, w591) -> (w599:bool[])
                        n211 = Equal?(x=w585, y=1.0) -> (x = y?=w575:bool)
                        n212 = Search 1D Array(1D array=w599, element=TRUE) -> (index of element=w597:i32)  [unwired: 1 in]
                        n213 = case shown="True" w575 {
                          tunnel: w597 -> [w607 _]
                          tunnel: [w606 w619] -> w593
                          tunnel: [w605 w622] -> w592
                          tunnel: w580 -> [w604 w620]
                          tunnel: w570 -> [_ w621]
                          tunnel: w569 -> [_ w618]
                          frame False {
                            n214 = case shown="3" w607 {
                              tunnel: [w609 w610 w612 w614 w617] -> w606
                              tunnel: w604 -> [w609 w610 w612 w614 w617]
                              tunnel: [u16 0 ("I/P") u16 3 ("I/P") u16 1 ("I/P") u16 4 ("I/P") u16 5 ("I/P")] -> w605
                              frame -1, Default {
                              }
                              frame 0 {
                              }
                              frame 1 {
                              }
                              frame 2 {
                              }
                              frame 3 {
                              }
                            }
                          }
                          frame True {
                            n215 = case shown="False" w621 {
                              tunnel: [w626 u16 1 ("I/P")] -> w622
                              tunnel: w620 -> [w625 w635]
                              tunnel: [w624 w635] -> w619
                              tunnel: w618 -> [w623 _]
                              frame False {
                                n216 = case shown="False" w623 {
                                tunnel: [u16 5 ("I/P") u16 1 ("I/P")] -> w626
                                tunnel: w625 -> [w628 w634]
                                tunnel: [w627 w634] -> w624
                                frame False {
                                n217 = global write "Global 1.vi" "RECHECK RESULT OK"(TRUE ("RECHECK RESULT OK")) -> ()
                                n218 = call "SEND RECHECK ABORT BUTTON.vi"("Enum"=enum16{"Read", "Write"}."Write", "error in (no error)"=w628, "Array"=u16[] [0]) -> ("error out"=w627:errorcluster)  [unwired: 7 in, 1 out]
                                }
                                frame True {
                                }
                                }
                              }
                              frame True {
                              }
                            }
                          }
                        }
                      }
                    }
                  }
                  frame True {
                    "OP40 BARCODE STRING EMPRTY" <- w639
                  }
                }
                n219 = call "PADMINI_AUTO_BARCODE_STATUS3.vi"("Enum"=enum16{"Read", "Write"}."Write", "error in (no error)"=w544, "I/P"=w542) -> ("error out"=w543:errorcluster)  [unwired: 7 in, 1 out]
              }
              frame True {
                n220 = call "PADMINI_AUTO_BARCODE_STATUS3.vi"("Enum"=enum16{"Read", "Write"}."Write", "error in (no error)"=w642, "I/P"=u16 1) -> ("error out"=w641:errorcluster)  [unwired: 7 in, 1 out]
              }
            }
            n221 = flat-sequence {
              tunnel: [w534] -> w522
              tunnel: w523 -> [w534]
              frame #0 {
                n222 = local write "OP40 BARCODE STRING EMPRTY"(FALSE) -> ()
                n223 = global write "DATA LOG.vi" "scan op 40"(TRUE ("scan op 40")) -> ()
                n224 = global write "DATA LOG.vi" "ST 3 STRING 2"("" ("ST 3 STRING 2")) -> ()
                n225 = global write "DATA LOG.vi" "op 40"(0 ("op 30")) -> ()
              }
            }
          }
          frame "SCAN4" {
            # "AC300711701GGN/PRCV241221045"
            # "Barcode Status\n0-Ideal, \n1-Ok, 2-Nok, 3-Prev Station Not Done,\n4-Prev Station Nok,\n5- Already Done"
            n226 = case shown="False" w651 {
              tunnel: w655 -> [w697 w833]
              tunnel: w654 -> [w681 w832]
              tunnel: w653 -> [w696 _]
              tunnel: [w687 w831] -> w649
              tunnel: [w689 w833] -> w652
              tunnel: w648 -> [w677 w828]
              tunnel: [w676 w828] -> w647
              tunnel: [w663 w827] -> w646
              tunnel: w645 -> [w668 w827]
              frame False {
                # "0 = IF STATION 1 RESULT IS EMPTY\n1 = IF STATION 1 RESULT IS TRUE IS (LOGGED)\n       AND STATION 2 RESULT IS EMPTY (NOT LOGGED YET)\n2 = IF STATION 1 DATA IS LODDED BUT ITS FALSE(NOK)\n3 = IF STATION 2 RESULT IS STILL EMPTY ( YET NOT LOGGED)"
                # "STATION 4 BARCODE STRING"
                n227 = global read "DATA LOG.vi" "ST 4 STRING 3"() -> (w671:string)
                "scanner value" <- w671
                n228 = Empty String/Path?(string/path=w671) -> (empty?=w673:bool)
                n229 = call "PADMINI_AUTO_BARCODE_STRING4.vi"("Enum"=enum16{"Read", "Write"}."Read", "error in (no error)"=w681) -> ("error out"=w680:errorcluster)  [unwired: 8 in, 1 out]
                n230 = Not(x=w673) -> (.not. x?=w674:bool)
                n231 = call <vilib>:"Trim Whitespace.vi"("string"=w671) -> ("trimmed string"=w663:string)  [unwired: 1 in]
                n232 = disable-structure shown="Enabled" {
                  disable-tunnel: "" -> [w825 _]
                  disable-tunnel: [w824 _] -> w682
                  disable-tunnel: w663 -> [w819 _]
                  disable-tunnel: [w820 TRUE] -> w675
                  frame Enabled {
                    n233 = global read "Global 1.vi" "BARCODE RECIPE"() -> (w818:string)
                    n234 = Match Pattern(string=w819, regular expression=w818) -> (match substring=w823:string)  [unwired: 1 in, 3 out]
                    n235 = String Length(string=w818) -> (length=w822:i32)
                    n236 = String Length(string=w823) -> (length=w821:i32)
                    n237 = Equal?(x=w819, y=w825) -> (x = y?=w824:bool)
                    n238 = Equal?(x=w822, y=w821) -> (x = y?=w820:bool)
                  }
                  frame Disabled {
                  }
                }
                n239 = Equal?(x=w668, y=w663) -> (x = y?=w667:bool)
                n240 = call-poly <userlib>:"Data Changed__ogtk.vi"("String"=w671) -> ("Changed"=w672:bool)
                n241 = Equal?(x=w663, y="ERROR") -> (x = y?=w665:bool)
                n242 = And(x=w672, y=w674) -> (x .and. y?=w670:bool)
                n243 = global write "Global 1.vi" "OP 60 BARCODE"(w663) -> ()
                n244 = local read "OP 60"() -> (w684:T7)
                n245 = Bundle By Name(cluster=w684, "BARCODE"=w663) -> (w678:T7)
                n246 = String To Byte Array(string=w663) -> (unsigned byte array=w679:u8[])
                n247 = Or(x=w667, y=w665) -> (x .or. y?=w664:bool)
                n248 = Format Into String(format string="where BARCODE='%s'", w663) -> (resulting string=w692:string)  [unwired: 2 in, 1 out]
                n249 = Not(x=w670) -> (.not. x?=w669:bool)
                n250 = global write "DATA LOG.vi" "string to bye array"(w679) -> ()
                n251 = global write "DATA LOG.vi" "test barcode"(w663) -> ()
                n252 = call <vilib>:"DB Tools Select Data.vi"("condition"=w692, "error in (no error)"=w680, "columns"=string[] ["BARCODE", "ST3_RESULT", "ST4_RESULT"], "table"=w696, "connection reference"=w697) -> ("error out"=w691:errorcluster, "data"=w690:variant[][], "connection reference out"=w689:T13)  [unwired: 1 in]
                n253 = local write "OP 61"(w678) -> ()
                n254 = local write "OP 60"(w678) -> ()
                n255 = case shown="False" w664 {
                  tunnel: w691 -> [w707 w815]
                  tunnel: w690 -> [w706 _]
                  tunnel: [w705 w814] -> w688
                  tunnel: [w704 u16 2 ("I/P")] -> w685
                  tunnel: w682 -> [w703 _]
                  tunnel: w677 -> [w702 w816]
                  tunnel: [w701 w816] -> w676
                  tunnel: w675 -> [w700 _]
                  tunnel: w669 -> [w699 _]
                  tunnel: w663 -> [w698 _]
                  frame False {
                    n256 = case shown="True" w703 {
                      selector: w703 -> [_ w807]
                      tunnel: w707 -> [w716 w806]
                      tunnel: w706 -> [w715 _]
                      tunnel: [w714 w805] -> w705
                      tunnel: [w713 u16 2 ("I/P")] -> w704
                      tunnel: w698 -> [w712 _]
                      tunnel: w702 -> [w711 w803]
                      tunnel: [w710 w803] -> w701
                      tunnel: w700 -> [w709 _]
                      tunnel: w699 -> [w708 _]
                      frame False {
                        n257 = case shown="True" w709 {
                          tunnel: w716 -> [w717 w758]
                          tunnel: w715 -> [_ w757]
                          tunnel: [w717 w747] -> w714
                          tunnel: [u16 2 ("I/P") w746] -> w713
                          tunnel: w712 -> [_ w739]
                          tunnel: w711 -> [w719 w738]
                          tunnel: [w719 w737] -> w710
                          tunnel: w708 -> [_ _]
                          frame False {
                          }
                          frame True {
                            n258 = call "PADMINI_varient_to_data.vi"("error in (no error)"=w758, "data"=w757) -> ("error out"=w727:errorcluster, "Array"=w748:string[][])  [unwired: 8 in]
                            n259 = Index Array(array=w748, index (row) #1=0 ("index (row)"), index (col) #1=1 ("disabled index (col)"), index (row) #2=0 ("index (row)"), index (col) #2=2 ("disabled index (col)")) -> (element #1=w729:string, element #2=w722:string)
                            n260 = call <vilib>:"Clear Errors.vi"("error in (no error)"=w727) -> ("error out"=w726:errorcluster)  [unwired: 5 in, 1 out]
                            n261 = Not Equal?(x=w729, y="OK") -> (x != y?=w755:bool)
                            n262 = Equal?(x=w729, y="OK") -> (x = y?=w751:bool)
                            n263 = Empty String/Path?(string/path=w729) -> (empty?=w756:bool)
                            n264 = Empty String/Path?(string/path=w722) -> (empty?=w749:bool)
                            n265 = call "READ OP60 RECHECK BIT.vi"("Enum"=enum16{"Read", "Write"}."Read", "error in (no error)"=w726) -> ("error out"=w721:errorcluster, "Input 2"=w735:dbl[])  [unwired: 8 in]
                            n266 = And(x=w751, y=w749) -> (x .and. y?=w750:bool)
                            n267 = Not(x=w749) -> (.not. x?=w745:bool)
                            n268 = Equal?(x=w722, y="NOK") -> (x = y?=w724:bool)
                            n269 = Equal?(x=w722, y="Aborted") -> (x = y?=w723:bool)
                            n270 = Index Array(array=w735, index=0) -> (element=w733:dbl)
                            n271 = Build Array(w756, w750, w755, w745) -> (w754:bool[])
                            n272 = Equal?(x=w733, y=1.0) -> (x = y?=w731:bool)
                            n273 = Search 1D Array(1D array=w754, element=TRUE) -> (index of element=w752:i32)  [unwired: 1 in]
                            n274 = call <vilib>:"Clear Errors.vi"("error in (no error)"=w721) -> ("error out"=w720:errorcluster)  [unwired: 5 in, 1 out]
                            n275 = case shown="True" w731 {
                              tunnel: w752 -> [w765 _]
                              tunnel: w720 -> [w764 w786]
                              tunnel: [w763 w785] -> w747
                              tunnel: [w762 w788] -> w746
                              tunnel: w739 -> [w761 _]
                              tunnel: w738 -> [w760 w787]
                              tunnel: [w759 w787] -> w737
                              tunnel: w724 -> [_ w784]
                              tunnel: w723 -> [_ w783]
                              frame False {
                                n276 = case shown="2" w765 {
                                tunnel: [w768 w770 w775 w778 w782] -> w763
                                tunnel: w764 -> [w768 w770 w775 w778 w782]
                                tunnel: [u16 2 ("I/P") u16 3 ("I/P") u16 1 ("I/P") u16 4 ("I/P") u16 5 ("I/P")] -> w762
                                tunnel: w761 -> [_ _ w774 _ _]
                                tunnel: w760 -> [w766 w769 w773 w777 w780]
                                tunnel: [w766 w769 w772 w777 w780] -> w759
                                frame -1 {
                                }
                                frame 0 {
                                }
                                frame 1, Default {
                                n277 = Build Array (concatenate)(w773, w774) -> (w772:string[])
                                }
                                frame 2 {
                                }
                                frame 3 {
                                }
                                }
                              }
                              frame True {
                                n278 = case shown="False" w784 {
                                tunnel: [w792 u16 1 ("I/P")] -> w788
                                tunnel: [w790 w802] -> w785
                                tunnel: w786 -> [w791 w802]
                                tunnel: w783 -> [w789 _]
                                frame False {
                                n279 = case shown="True" w789 {
                                tunnel: [u16 5 ("I/P") u16 1 ("I/P")] -> w792
                                tunnel: w791 -> [w794 w799]
                                tunnel: [w793 w799] -> w790
                                frame False {
                                n280 = global write "Global 1.vi" "RECHECK RESULT OK"(TRUE ("RECHECK RESULT OK")) -> ()
                                n281 = call "RESET RECHECK OP60 BIT.vi"("Enum"=enum16{"Read", "Write"}."Write", "error in (no error)"=w794, "Array"=u16[] [0]) -> ("error out"=w793:errorcluster)  [unwired: 7 in, 1 out]
                                }
                                frame True {
                                }
                                }
                                }
                                frame True {
                                }
                                }
                              }
                            }
                          }
                        }
                      }
                      frame True {
                        n282 = disable-structure shown="Enabled" {
                          disable-tunnel: w806 -> [w811 w813]
                          disable-tunnel: [w810 w812] -> w805
                          frame Disabled {
                            n283 = call "PADMINI_AUTO_BARCODE_STATUS4.vi"("Enum"=enum16{"Read", "Write"}."Write", "error in (no error)"=w811, "I/P"=u16 2) -> ("error out"=w810:errorcluster)  [unwired: 7 in, 1 out]
                          }
                          frame Enabled {
                            n284 = call <vilib>:"Clear Errors.vi"("error in (no error)"=w813) -> ("error out"=w812:errorcluster)  [unwired: 5 in, 1 out]
                          }
                        }
                        "Boolean 5" <- w807
                      }
                    }
                  }
                  frame True {
                    n285 = call <vilib>:"Clear Errors.vi"("error in (no error)"=w815) -> ("error out"=w814:errorcluster)  [unwired: 5 in, 1 out]
                  }
                }
                n286 = call "PADMINI_AUTO_BARCODE_STATUS4.vi"("Enum"=enum16{"Read", "Write"}."Write", "error in (no error)"=w688, "I/P"=w685) -> ("error out"=w687:errorcluster)  [unwired: 7 in, 1 out]
                "PRIVIOUS DATA" <- w668
              }
              frame True {
                n287 = call "PADMINI_AUTO_BARCODE_STATUS4.vi"("Enum"=enum16{"Read", "Write"}."Write", "error in (no error)"=w832, "I/P"=u16 1) -> ("error out"=w831:errorcluster)  [unwired: 7 in, 1 out]
              }
            }
            n288 = flat-sequence {
              tunnel: [w660] -> w650
              tunnel: w649 -> [w661]
              frame #0 {
                n289 = call "PADMINI_AUTO_BARCODE_STRING4.vi"("Enum"=enum16{"Read", "Write"}."Write", "error in (no error)"=w661, "Input"="" ("ST 4 STRING 3")) -> ("error out"=w660:errorcluster)  [unwired: 7 in, 1 out]
                n290 = local write "Boolean 5"(TRUE ("Boolean 5")) -> ()
                n291 = global write "DATA LOG.vi" "scan op 60"(TRUE ("scan op 60")) -> ()
              }
            }
          }
          frame "DATALOG2" {
            w835 = T14 2 items=["no dialog", "OK message", "continue or stop message", "OK message + warnings", "continue/stop + warnings"] ("type of dialog (OK msg:1)")
            # "ST2_REAL_DATA\nST2_BOOL_DATA\nDATE\nSHIFT"
            # "datalog of st 2"
            n292 = local read "STATION-2 2"() -> (w869:T3)
            n293 = call "PADMINI_AUTO_CYCLE STATE2.vi"("Enum"=enum16{"Read", "Write"}."Read", "error in (no error)"=w841) -> ("error out"=w840:errorcluster, "Input 2"=w844:u16[])  [unwired: 8 in]
            n294 = Unbundle By Name(w869) -> ("BARCODE"=w855:string, "OK PART"=w865:dbl, "NOK PART"=w864:dbl, "TOTAL"=w863:dbl, "CYCLE TIME"=w868:dbl, "PARAMETER 1"=w867:dbl, "PARAMETER 2"=w866:dbl, "SCANNER"=w862:bool, "CYCLE STATUS"=w861:bool, "PARAMETER 1"=w860:bool, "PARAMETER 2"=w859:bool, "CYCLE RESULT"=w847:bool)  [unwired: 9 out]
            n295 = Index Array(array=w844, index=2) -> (element=w843:u16)
            n296 = case shown="3" w843 {
              tunnel: ["" "OK" "NOK" "Aborted"] -> w842
              frame 0 {
              }
              frame 1, Default {
              }
              frame 2 {
              }
              frame 3 {
              }
            }
            n297 = Build Array(w865, w864, w863, w868, w867, w866) -> (w854:dbl[])
            n298 = Build Array(w862, w861, w860, w859) -> (w853:bool[])
            n299 = case shown="False" w857 {
              tunnel: w858 -> [w891 w905]
              tunnel: w840 -> [w890 w904]
              tunnel: [w889 w903] -> w852
              tunnel: [w888 w902] -> w837
              tunnel: w856 -> [w887 _]
              tunnel: w855 -> [w881 _]
              tunnel: w854 -> [w884 w898]
              tunnel: w853 -> [w879 w897]
              tunnel: w847 -> [_ w893]
              tunnel: w842 -> [w877 w892]
              frame False {
                n300 = local read "SHIFT"() -> (w886:string)
                n301 = call "PADMINI_SHIFT_DATE.vi"("SHIFT"=w886) -> ("date/time string"=w885:string)  [unwired: 10 in]
                n302 = Bundle("SHIFT"=w886, "date/time string"=w885, w884, w879, w877) -> (w878:T17)  [unwired: 1 in]
                n303 = To Variant(anything=w878) -> ()  [unwired: 1 out]
                n304 = Format Into String(format string="where BARCODE='%s'", w881) -> (resulting string=w880:string)  [unwired: 2 in, 1 out]
                n305 = call <vilib>:"DB Tools Update Data.vi"("condition"=w880, "data"=w878, "error in (no error)"=w890, "columns"=string[] ["SHIFT", "DATE", "ST2_REAL_DATA", "ST2_BOOL_DATA", "ST2_RESULT"], "table"=w887, "connection reference"=w891) -> ("error out"=w888:errorcluster, "connection reference out"=w889:T13)  [unwired: 4 in]
              }
              frame True {
                n306 = local read "SHIFT"() -> (w900:string)
                n307 = call "PADMINI_SHIFT_DATE.vi"("SHIFT"=w900) -> ("date/time string"=w899:string)  [unwired: 10 in]
                n308 = Bundle("SHIFT"=w900, "date/time string"=w899, w898, w897, "CYCLE RESULT"=w893, w892) -> (w896:T16)  [unwired: 1 in]
                n309 = To Variant(anything=w896) -> (Variant=w895:variant)
                n310 = call <vilib>:"DB Tools Insert Data.vi"("data"=w895, "error in (no error)"=w904, "columns"=string[] ["SHIFT", "DATE", "ST2_REAL_DATA", "ST2_BOOL_DATA", "ST2_RESULT", "RESULT"], "table"="ST2_REPORT", "connection reference"=w905) -> ("error out"=w902:errorcluster, "connection reference out"=w903:T13)  [unwired: 5 in]
              }
            }
            n311 = call <vilib>:"Simple Error Handler.vi"("type of dialog (OK msg:1)"=w835, "error in (no error)"=w837) -> ("error out"=w838:errorcluster)  [unwired: 3 in, 4 out]
            n312 = call <vilib>:"Clear Errors.vi"("error in (no error)"=w838) -> ("error out"=w836:errorcluster)  [unwired: 5 in, 1 out]
            n313 = flat-sequence {
              tunnel: [w875] -> w848
              tunnel: w849 -> [w875]
              frame #0 {
                n314 = global write "DATA LOG.vi" "DATA LOG RESET 2"(TRUE ("DATA LOG RESET")) -> ()
              }
            }
            n315 = call "PADMINI_AUTO_DATALOG_DONE2.vi"("Enum"=enum16{"Read", "Write"}."Write", "error in (no error)"=w836, "I/P"=u16 2) -> ("error out"=w849:errorcluster)  [unwired: 7 in, 1 out]
          }
          frame "DATALOG3" {
            w908 = T14 2 items=["no dialog", "OK message", "continue or stop message", "OK message + warnings", "continue/stop + warnings"] ("type of dialog (OK msg:1)")
            # "ST3_REAL_DATA\nST3_BOOL_DATA\nDATE\nSHIFT"
            # "datalog of st 3"
            n316 = local read "STATION-3 2"() -> (w951:T3)
            n317 = call "PADMINI_AUTO_CYCLE STATE3.vi"("Enum"=enum16{"Read", "Write"}."Read", "error in (no error)"=w915) -> ("error out"=w914:errorcluster, "Input 2"=w916:u16[])  [unwired: 8 in]
            n318 = Unbundle By Name(w951) -> ("BARCODE"=w927:string, "OK PART"=w942:dbl, "NOK PART"=w941:dbl, "TOTAL"=w940:dbl, "CYCLE TIME"=w950:dbl, "PARAMETER 1"=w949:dbl, "PARAMETER 2"=w948:dbl, "PARAMETER 3"=w947:dbl, "PARAMETER 4"=w946:dbl, "PARAMETER 5"=w945:dbl, "PARAMETER 6"=w944:dbl, "PARAMETER 7"=w943:dbl, "SCANNER"=w939:bool, "CYCLE STATUS"=w938:bool, "PARAMETER 1"=w937:bool, "PARAMETER 2"=w936:bool, "PARAMETER 3"=w935:bool, "PARAMETER 4"=w934:bool, "PARAMETER 5"=w933:bool, "PARAMETER 6"=w932:bool, "PARAMETER 7"=w931:bool, "CYCLE RESULT"=w920:bool)  [unwired: 4 out]
            n319 = Index Array(array=w916, index=2) -> (element=w918:u16)
            n320 = case shown="2" w918 {
              tunnel: ["" "OK" "NOK" "Aborted"] -> w913
              frame 0 {
              }
              frame 1, Default {
              }
              frame 2 {
              }
              frame 3 {
              }
            }
            n321 = Build Array(w942, w941, w940, w950, w949, w948, w947, w946, w945, w944, w943) -> (w926:dbl[])
            n322 = Build Array(w939, w938, w937, w936, w935, w934, w933, w932, w931) -> (w925:bool[])
            n323 = case shown="True" w929 {
              tunnel: w930 -> [w973 w985]
              tunnel: w914 -> [w972 w984]
              tunnel: [w971 w983] -> w924
              tunnel: [w970 w982] -> w909
              tunnel: w928 -> [w969 _]
              tunnel: w927 -> [w963 _]
              tunnel: w926 -> [w966 w978]
              tunnel: w925 -> [w961 w977]
              tunnel: w920 -> [_ _]
              tunnel: w913 -> [w960 w975]
              frame False {
                n324 = local read "SHIFT"() -> (w968:string)
                n325 = call "PADMINI_SHIFT_DATE.vi"("SHIFT"=w968) -> ("date/time string"=w967:string)  [unwired: 10 in]
                n326 = Bundle("SHIFT"=w968, "date/time string"=w967, w966, w961, w960) -> (w959:T17)  [unwired: 1 in]
                n327 = Format Into String(format string="where BARCODE='%s'", w963) -> (resulting string=w962:string)  [unwired: 2 in, 1 out]
                n328 = To Variant(anything=w959) -> ()  [unwired: 1 out]
                n329 = call <vilib>:"DB Tools Update Data.vi"("condition"=w962, "data"=w959, "error in (no error)"=w972, "columns"=string[] ["SHIFT", "DATE", "ST3_REAL_DATA", "ST3_BOOL_DATA", "ST3_RESULT"], "table"=w969, "connection reference"=w973) -> ("error out"=w970:errorcluster, "connection reference out"=w971:T13)  [unwired: 4 in]
              }
              frame True {
                n330 = local read "SHIFT"() -> (w980:string)
                n331 = call "PADMINI_SHIFT_DATE.vi"("SHIFT"=w980) -> ("date/time string"=w979:string)  [unwired: 10 in]
                n332 = Bundle("SHIFT"=w980, "date/time string"=w979, w978, w977, w975) -> (w974:T17)  [unwired: 1 in]
                n333 = To Variant(anything=w974) -> ()  [unwired: 1 out]
                n334 = call <vilib>:"DB Tools Insert Data.vi"("data"=w974, "error in (no error)"=w984, "columns"=string[] ["SHIFT", "DATE", "ST3_REAL_DATA", "ST3_BOOL_DATA", "ST3_RESULT", "RESULT"], "table"="ST3_REPORT", "connection reference"=w985) -> ("error out"=w982:errorcluster, "connection reference out"=w983:T13)  [unwired: 5 in]
              }
            }
            n335 = call <vilib>:"Simple Error Handler.vi"("type of dialog (OK msg:1)"=w908, "error in (no error)"=w909) -> ("error out"=w910:errorcluster)  [unwired: 3 in, 4 out]
            n336 = call <vilib>:"Clear Errors.vi"("error in (no error)"=w910) -> ("error out"=w907:errorcluster)  [unwired: 5 in, 1 out]
            n337 = flat-sequence {
              tunnel: [w957] -> w921
              tunnel: w922 -> [w957]
              frame #0 {
                n338 = global write "DATA LOG.vi" "DATA LOG RESET 3"(TRUE ("DATA LOG RESET")) -> ()
              }
            }
            n339 = call "PADMINI_AUTO_DATALOG_DONE3.vi"("Enum"=enum16{"Read", "Write"}."Write", "error in (no error)"=w907, "I/P"=u16 2) -> ("error out"=w922:errorcluster)  [unwired: 7 in, 1 out]
          }
          frame "DATALOG4" {
            w1004 = 0 ("disabled index (row)")
            w1021 = T14 2 items=["no dialog", "OK message", "continue or stop message", "OK message + warnings", "continue/stop + warnings"] ("type of dialog (OK msg:1)")
            # "ST4_REAL_DATA\nST4_BOOL_DATA\nDATE\nSHIFT"
            # "datalog of st 4"
            n340 = disable-structure shown="Enabled" {
              frame Disabled {
                n341 = call "barcode st4.vi"("Enum"=enum16{"Read", "Write"}."Read") -> ()  [unwired: 9 in, 2 out]
              }
              frame Enabled {
              }
            }
            n342 = local read "STATION-4 2"() -> (w1068:T3)
            n343 = Unbundle By Name(w1068) -> ("BARCODE"=w1028:string, "OK PART"=w1062:dbl, "NOK PART"=w1061:dbl, "TOTAL"=w1060:dbl, "CYCLE TIME"=w1067:dbl, "PARAMETER 1"=w1066:dbl, "PARAMETER 2"=w1065:dbl, "PARAMETER 3"=w1064:dbl, "PARAMETER 4"=w1063:dbl, "SCANNER"=w1059:bool, "CYCLE STATUS"=w1058:bool, "PARAMETER 1"=w1057:bool, "PARAMETER 2"=w1056:bool, "PARAMETER 3"=w1055:bool, "PARAMETER 4"=w1054:bool, "PARAMETER 5"=w1053:bool, "PARAMETER 6"=w1052:bool, "PARAMETER 7"=w1051:bool, "PARAMETER 8"=w1050:bool, "PARAMETER 9"=w1049:bool, "PARAMETER 10"=w1048:bool, "CYCLE RESULT"=w1039:bool)  [unwired: 7 out]
            n344 = call "PADMINI_AUTO_CYCLE STATE4.vi"("Enum"=enum16{"Read", "Write"}."Read", "error in (no error)"=w1024) -> ("error out"=w1014:errorcluster, "Input 2"=w1034:u16[])  [unwired: 8 in]
            n345 = Index Array(array=w1034, index=2) -> (element=w1037:u16)
            n346 = Index Array(array=w1032) -> (element=w1033:string)  [unwired: 1 in]
            n347 = case shown="0" w1037 {
              tunnel: ["" "OK" "NOK" "Aborted"] -> w1036
              frame 0 {
              }
              frame 1, Default {
              }
              frame 2 {
              }
              frame 3 {
              }
            }
            n348 = call <vilib>:"Trim Whitespace.vi"("string"=w1033) -> ("trimmed string"=w1027:string)  [unwired: 1 in]
            n349 = call <vilib>:"Trim Whitespace.vi"("string"=w1028) -> ("trimmed string"=w1026:string)  [unwired: 1 in]
            n350 = call <vilib>:"Clear Errors.vi"("error in (no error)"=w1024) -> ("error out"=w1023:errorcluster)  [unwired: 5 in, 1 out]
            n351 = Build Array(w1062, w1061, w1060, w1067, w1066, w1065, w1064, w1063) -> (w1046:dbl[])
            "LOG DATA 2" <- w1046
            n352 = Build Array(w1059, w1058, w1057, w1056, w1055, w1054, w1053, w1052, w1051, w1050, w1049, w1048) -> (w1045:bool[])
            n353 = Delete From Array(array=w1032, length=1, index=0) -> (array with subset deleted=w1029:string[])  [unwired: 1 out]
            n354 = disable-structure shown="Enabled" {
              disable-tunnel: w1027 -> [w1074 _]
              disable-tunnel: w1026 -> [w1073 _]
              disable-tunnel: [w1072 w1079] -> w1010
              disable-tunnel: w1023 -> [_ w1078]
              disable-tunnel: [_ w1077] -> w1025
              frame Disabled {
                n355 = Empty String/Path?(string/path=w1074) -> (empty?=w1075:bool)
                n356 = Select(t=w1073, s=w1075, f=w1074) -> (s? t:f=w1072:string)
              }
              frame Enabled {
                n357 = call "REAS BARCODE STRING.vi"("error in (no error)"=w1078, "Enum"=enum16{"Read", "Write"}."Read") -> ("error out"=w1077:errorcluster, "Input 2"=w1079:string)  [unwired: 8 in]
                "Input 3" <- w1079
              }
            }
            n358 = Format Into String(format string="where BARCODE='%s'", w1010) -> (resulting string=w1009:string)  [unwired: 2 in, 1 out]
            n359 = call <vilib>:"DB Tools Select Data.vi"("condition"=w1009, "error in (no error)"=w1014, "columns"=string[] ["SHIFT", "DATE", "ST4_REAL_DATA", "ST4_BOOL_DATA", "ST4_RESULT"], "table"=w1008, "connection reference"=w1013) -> ("error out"=w1017:errorcluster, "data"=w1016:variant[][], "connection reference out"=w1012:T13)  [unwired: 1 in]
            n360 = Variant To Data(error in=w1017, type=string[][] [], Variant=w1016) -> (data=w1006:string[][], error out=w991:errorcluster)
            n361 = Index Array(array=w1006, index (row) #1=w1004, index (col) #1=2 ("disabled index (col)"), index (row) #2=w1004, index (col) #2=3 ("disabled index (col)"), index (row) #3=w1004, index (col) #3=4 ("disabled index (col)")) -> (element #1=w994:string, element #3=w1001:string)  [unwired: 1 out]
            n362 = Unflatten From String(type=dbl[] [] ("subarray"), binary string=w994, error in (no error)=w991) -> (value=w997:dbl[], error out=w999:errorcluster)  [unwired: 2 in, 1 out]
            n363 = call <vilib>:"Clear Errors.vi"("error in (no error)"=w999) -> ("error out"=w990:errorcluster)  [unwired: 5 in, 1 out]
            n364 = Delete From Array(array=w997, length=3, index=0) -> (array with subset deleted=w993:dbl[])  [unwired: 1 out]
            "array w/ subset deleted" <- w993
            n365 = Equal?(x=w1001, y="OK") -> (x = y?=w988:bool)
            n366 = Search 1D Array(1D array=w993, element=0.0) -> (index of element=w989:i32)  [unwired: 1 in]
            n367 = case shown="-1" w989 {
              tunnel: [FALSE TRUE] -> w987
              frame 0, Default {
              }
              frame -1 {
              }
            }
            n368 = And(x=w988, y=w987) -> (x .and. y?=w986:bool)
            n369 = case shown="False" w1047 {
              tunnel: w1012 -> [w1104 w1126]
              tunnel: w990 -> [_ w1125]
              tunnel: [w1103 w1124] -> w1044
              tunnel: [w1102 w1123] -> w1020
              tunnel: w1008 -> [w1101 _]
              tunnel: w1010 -> [w1091 _]
              tunnel: w1046 -> [w1098 w1119]
              tunnel: w1045 -> [w1094 w1118]
              tunnel: w1039 -> [_ _]
              tunnel: w1036 -> [w1093 w1116]
              tunnel: w1025 -> [w1089 _]
              tunnel: w986 -> [w1088 _]
              frame False {
                n370 = local read "SHIFT"() -> (w1100:string)
                n371 = call <vilib>:"Trim Whitespace.vi"("string"=w1091) -> ("trimmed string"=w1090:string)  [unwired: 1 in]
                "LOG DATA" <- w1090
                n372 = call "PADMINI_SHIFT_DATE.vi"("SHIFT"=w1100) -> ("date/time string"=w1099:string)  [unwired: 10 in]
                n373 = Bundle("SHIFT"=w1100, "date/time string"=w1099, w1098, w1094, w1093) -> (w1092:T17)  [unwired: 1 in]
                n374 = To Variant(anything=w1092) -> ()  [unwired: 1 out]
                n375 = Format Into String(format string="where BARCODE='%s'", w1090) -> (resulting string=w1095:string)  [unwired: 2 in, 1 out]
                "resulting string" <- w1095
                n376 = case shown="False" w1088 {
                  tunnel: w1104 -> [w1112 w1113]
                  tunnel: [w1111 w1113] -> w1103
                  tunnel: [w1110 w1114] -> w1102
                  tunnel: w1101 -> [w1109 _]
                  tunnel: string[] ["SHIFT", "DATE", "ST4_REAL_DATA", "ST4_BOOL_DATA", "ST4_RESULT"] -> [w1108 _]
                  tunnel: w1095 -> [w1107 _]
                  tunnel: w1092 -> [w1106 _]
                  tunnel: w1089 -> [w1105 w1114]
                  frame False {
                    n377 = call <vilib>:"DB Tools Update Data.vi"("condition"=w1107, "data"=w1106, "error in (no error)"=w1105, "columns"=w1108, "table"=w1109, "connection reference"=w1112) -> ("error out"=w1110:errorcluster, "connection reference out"=w1111:T13)  [unwired: 4 in]
                  }
                  frame True {
                  }
                }
                "error out 5" <- w1102
              }
              frame True {
                n378 = local read "SHIFT"() -> (w1121:string)
                n379 = call "PADMINI_SHIFT_DATE.vi"("SHIFT"=w1121) -> ("date/time string"=w1120:string)  [unwired: 10 in]
                n380 = Bundle("SHIFT"=w1121, "date/time string"=w1120, w1119, w1118, w1116) -> (w1115:T17)  [unwired: 1 in]
                n381 = To Variant(anything=w1115) -> ()  [unwired: 1 out]
                n382 = call <vilib>:"DB Tools Insert Data.vi"("data"=w1115, "error in (no error)"=w1125, "columns"=string[] ["SHIFT", "DATE", "ST4_REAL_DATA", "ST4_BOOL_DATA", "ST4_RESULT", "RESULT"], "table"="ST4_REPORT", "connection reference"=w1126) -> ("error out"=w1123:errorcluster, "connection reference out"=w1124:T13)  [unwired: 5 in]
              }
            }
            n383 = call <vilib>:"Simple Error Handler.vi"("type of dialog (OK msg:1)"=w1021, "error in (no error)"=w1020) -> ("error out"=w1022:errorcluster)  [unwired: 3 in, 4 out]
            n384 = call <vilib>:"Clear Errors.vi"("error in (no error)"=w1022) -> ("error out"=w1019:errorcluster)  [unwired: 5 in, 1 out]
            n385 = flat-sequence {
              tunnel: [w1086] -> w1040
              tunnel: w1041 -> [w1086]
              frame #0 {
                n386 = global write "DATA LOG.vi" "DATA LOG RESET 4"(TRUE ("DATA LOG RESET")) -> ()
                n387 = local write "DATA"(FALSE ("Boolean 6")) -> ()
              }
            }
            n388 = call "PADMINI_AUTO_DATALOG_DONE4.vi"("Enum"=enum16{"Read", "Write"}."Write", "error in (no error)"=w1019, "I/P"=u16 2) -> ("error out"=w1041:errorcluster)  [unwired: 7 in, 1 out]
          }
          frame "BARCODE RECIPE" {
            w1133 = string[][] []
            w1143 = string[] ["BARCODE_RECIPE"] ("columns")
            w1136 = "BARCODE_RECIPE" ("table")
            # "NOT USED THIS CASE  AFTER TAHT LOGIC IS CHANGE  BARCODE RECIPE LOAD IN SETTING WINDOW"
            n389 = local read "BARCODE RECIPE"() -> (w1144:string)
            n390 = Format Into String(format string="WHERE BARCODE_RECIPE = '%s' ", w1144) -> (resulting string=w1142:string)  [unwired: 2 in, 1 out]
            n391 = call <vilib>:"DB Tools Select Data.vi"("condition"=w1142, "error in (no error)"=w1151, "columns"=w1143, "table"=w1136, "connection reference"=w1152) -> ("error out"=w1148:errorcluster, "data"=w1149:variant[][], "connection reference out"=w1145:T13)  [unwired: 1 in]
            n392 = Variant To Data(error in=w1148, type=w1133, Variant=w1149) -> (data=w1139:string[][], error out=w1146:errorcluster)
            n393 = Empty Array?(array=w1139) -> (empty?=w1147:bool)
            n394 = case shown="False" w1147 {
              tunnel: w1146 -> [w1153 w1162]
              tunnel: w1145 -> [w1154 w1161]
              tunnel: [w1154 w1160] -> w1137
              tunnel: [w1153 w1159] -> w1135
              tunnel: w1144 -> [_ w1158]
              tunnel: w1136 -> [_ w1156]
              tunnel: w1143 -> [_ w1155]
              tunnel: w1142 -> [_ _]
              frame False {
              }
              frame True {
                n395 = Bundle("BARCODE RECIPE"=w1158) -> (w1157:cluster{" BARCODE RECIPE":string})  [unwired: 1 in]
                n396 = call <vilib>:"DB Tools Insert Data.vi"("data"=w1157, "error in (no error)"=w1162, "columns"=w1155, "table"=w1156, "connection reference"=w1161) -> ("error out"=w1159:errorcluster, "connection reference out"=w1160:T13)  [unwired: 5 in]
              }
            }
            n397 = call <vilib>:"DB Tools Select Data.vi"("error in (no error)"=w1135, "table"=w1136, "connection reference"=w1137) -> ("error out"=w1130:errorcluster, "data"=w1132:variant[][], "connection reference out"=w1134:T13)  [unwired: 3 in]
            n398 = Variant To Data(error in=w1130, type=w1133, Variant=w1132) -> (data=w1131:string[][], error out=w1129:errorcluster)
            n399 = Index Array(array=w1131, index (col)=0 ("disabled index (col)")) -> (element=w1138:string[])  [unwired: 1 in]
            n400 = property on="BARCODE RECIPE" class="CmbBox"("Strings[]"=w1138) -> ()  [unwired: 2 in, 2 out]
          }
          frame "EMERGENCY STOP" {
          }
          frame "STOP" {
            n401 = global read "Global 1.vi" "BARCODE RECIPE"() -> (w1171:string)
            n402 = Bundle("BARCODE RECIPE"=w1171) -> (w1170:cluster{"BARCODE RECIPE":string})  [unwired: 1 in]
            n403 = call <vilib>:"DB Tools Update Data.vi"("data"=w1170, "error in (no error)"=w1176, "columns"=string[] ["PREVIOUS_LOADED_RECIPE"], "table"="BARCODE_RECIPE", "connection reference"=w1174) -> ("error out"=w1175:errorcluster, "connection reference out"=w1173:T13)  [unwired: 5 in]
          }
        }
      }
      frame Error {
        # "Return true in any case that should stop the loop."
      }
    }
    n404 = Wait (ms)(milliseconds to wait=u32 100) -> ()  [unwired: 1 out]
  }
  n405 = while {
    shift-right: [w1253] -> w102
    shift-left: w19 -> [w1185]
    shift-right: [w1254] -> w96
    shift-left: w100 -> [w1262]
    stop <- w1252 stop-if-true
    w1250 = enum16{"Read", "Write"}."Read" ("Enum")
    # "ST 4 Cycle start bit"
    # "ST 3 Cycle start bit"
    # "ST 2 Cycle start bit"
    # "Barcode Scan Data"
    # "Data Lock"
    n406 = global read "Global 1.vi" "PLC COMM"() -> (→"PLC COM.":bool)
    n407 = global read "Global 1.vi" "PLC 1"() -> (→"Boolean":bool)
    n408 = global read "Global 1.vi" "PLC 2"() -> (→"Boolean 2":bool)
    n409 = global read "Global 1.vi" "PLC 3"() -> (→"Boolean 3":bool)
    n410 = global read "Global 1.vi" "PLC 4"() -> (→"Boolean 4":bool)
    n411 = call <vilib>:"Clear Errors.vi"("error in (no error)"=w1185) -> ("error out"=w1184:errorcluster)  [unwired: 5 in, 1 out]
    n412 = call "READ EMERGENCY BIT.vi"("Enum"=enum16{"Read", "Write"}."Read", "error in (no error)"=w1184) -> ("Array Out"=w1191:dbl[])  [unwired: 8 in, 1 out]
    n413 = call "PADMINI_AUTO_CYCLE STATE2.vi"("Enum"=enum16{"Read", "Write"}."Read", "error in (no error)"=w1184) -> ("Input 2"=w1221:u16[])  [unwired: 8 in, 1 out]
    n414 = call "PADMINI_AUTO_CYCLE STATE3.vi"("Enum"=enum16{"Read", "Write"}."Read", "error in (no error)"=w1184) -> ("Input 2"=w1216:u16[])  [unwired: 8 in, 1 out]
    n415 = call "PADMINI_AUTO_CYCLE_BIT.vi"("Enum"=w1250, "error in (no error)"=w1184) -> ("Input 2"=w1249:u16[])  [unwired: 8 in, 1 out]
    n416 = call "PADMINI_AUTO_CYCLE_BIT2.vi"("Enum"=w1250, "error in (no error)"=w1184) -> ("Input 2"=w1246:u16[])  [unwired: 8 in, 1 out]
    n417 = call "PADMINI_AUTO_CYCLE_BIT3.vi"("Enum"=w1250, "error in (no error)"=w1184) -> ("Input 2"=w1244:u16[])  [unwired: 8 in, 1 out]
    n418 = call "PADMINI_AUTO_CYCLE_BIT4.vi"("Enum"=w1250, "error in (no error)"=w1184) -> ("Input 2"=w1245:u16[])  [unwired: 8 in, 1 out]
    n419 = call "PADMINI_AUTO_CYCLE STATE4.vi"("Enum"=enum16{"Read", "Write"}."Read", "error in (no error)"=w1184) -> ("Input 2"=w1212:u16[])  [unwired: 8 in, 1 out]
    n420 = Index Array(array=w1212, index=0) -> (element=w1211:u16)
    n421 = Index Array(array=w1216, index=0) -> (element=w1215:u16)
    n422 = Index Array(array=w1191) -> (element=w1190:dbl)  [unwired: 1 in]
    n423 = Index Array(array=w1221, index=0) -> (element=w1219:u16)
    n424 = Index Array(array=w1244, index #1=2 ("index"), index #2=1 ("index")) -> (element #2=w1227:u16)  [unwired: 1 out]
    n425 = Index Array(array=w1245, index #1=2 ("index"), index #2=1 ("index")) -> (element #2=w1187:u16)  [unwired: 1 out]
    n426 = Index Array(array=w1249, index #1=2 ("index"), index #2=1 ("index")) -> (element #1=w1237:u16, element #2=w1236:u16, element #3=w1223:u16)  [unwired: 1 in]
    n427 = Index Array(array=w1246, index #1=2 ("index"), index #2=1 ("index")) -> (element #2=w1235:u16)  [unwired: 1 out]
    n428 = global read "DATA LOG.vi" "op 40"() -> (w1208:i32)
    n429 = global read "DATA LOG.vi" "op 60"() -> (w1207:i32)
    n430 = global read "DATA LOG.vi" "op 30"() -> (w1209:i32)
    n431 = call "ST4 DATALOG.vi"("Numeric"=w1187) -> ("Boolean"=w1186:bool)  [unwired: 9 in, 1 out]
    "Boolean 6" <- w1186
    n432 = call "VALUE_CHANGE1.vi"("Numeric"=w1237) -> ("Boolean"=w1226:bool)  [unwired: 9 in, 1 out]
    n433 = call "VALUE_CHANGE - ST1_RESULT.vi"("Numeric"=w1236) -> ("Boolean"=w1200:bool)  [unwired: 9 in, 1 out]
    n434 = call "VALUE_CHANGE2.vi"("Numeric"=w1209) -> ("Boolean"=w1210:bool)  [unwired: 9 in, 1 out]
    n435 = call "VALUE_CHANGE - ST2_RESULT.vi"("Numeric"=w1235) -> ("Boolean"=w1234:bool)  [unwired: 9 in, 1 out]
    n436 = call "VALUE_CHANGE3.vi"("Numeric"=w1208) -> ("Boolean"=w1202:bool)  [unwired: 9 in, 1 out]
    n437 = call "VALUE_CHANGE - ST3_RESULT.vi"("Numeric"=w1227) -> ("Boolean"=w1233:bool)  [unwired: 9 in, 1 out]
    n438 = call "VALUE_CHANGE4.vi"("Numeric"=w1207) -> ("Boolean"=w1232:bool)  [unwired: 9 in, 1 out]
    n439 = call "VALUE_CHANGE - ST1_RESULT.vi"("Numeric"=w1223) -> ("Boolean"=w1225:bool)  [unwired: 9 in, 1 out]
    n440 = call "VALUE_CHANGE - ST1_RESULT.vi"("Numeric"=w1219) -> ("Boolean"=w1224:bool)  [unwired: 9 in, 1 out]
    n441 = call "VALUE_CHANGE - ST1_RESULT.vi"("Numeric"=w1215) -> ("Boolean"=w1206:bool)  [unwired: 9 in, 1 out]
    n442 = call "VALUE_CHANGE - ST1_RESULT.vi"("Numeric"=w1211) -> ("Boolean"=w1204:bool)  [unwired: 9 in, 1 out]
    n443 = call "VALUE_CHANGE - ST1_RESULT.vi"("Numeric"=w1190) -> ("Boolean"=w1188:bool)  [unwired: 9 in, 1 out]
    n444 = call <userlib>:"Boolean Trigger__ogtk.vi"("Boolean Input"=w1200) -> ("Rising Edge"=w1199:bool)  [unwired: 1 in, 1 out]
    n445 = call <userlib>:"Boolean Trigger__ogtk.vi"("Boolean Input"=w1202) -> ("Rising Edge"=w1201:bool)  [unwired: 1 in, 1 out]
    n446 = call "FIND TURE FOR AUTO.vi"("CYCLE START"="NEXT") -> ("Boolean"=w1196:bool)  [unwired: 8 in]
    n447 = call "FIND TURE FOR AUTO.vi"("CYCLE START"="Back") -> ("Boolean"=w1195:bool)  [unwired: 8 in]
    n448 = call <userlib>:"Boolean Trigger__ogtk.vi"("Boolean Input"=w1188) -> ("Rising Edge"=w1189:bool)  [unwired: 1 in, 1 out]
    n449 = call "FIND TURE FOR AUTO.vi"("CYCLE START"="Add Button") -> ("Boolean"=w1193:bool)  [unwired: 8 in]
    n450 = call <userlib>:"Boolean Trigger__ogtk.vi"("Boolean Input"=w1206) -> ("Rising Edge"=w1205:bool)  [unwired: 1 in, 1 out]
    n451 = call <userlib>:"Boolean Trigger__ogtk.vi"("Boolean Input"=w1204) -> ("Rising Edge"=w1203:bool)  [unwired: 1 in, 1 out]
    n452 = global write "Global 1.vi" "EMERGENCY STOP"(w1188) -> ()
    n453 = Build Array(w1226, w1199, w1210, w1234, w1201, w1233, w1232, w1186, w1225, w1224, w1205, w1203, w1196, w1195, w1193, w1189) -> (w1251:bool[])
    n454 = local read "Shift_change"() -> (w1260:bool)
    n455 = for {
      tunnel: w1251 -> [w1426] mode=indexing
      tunnel: [w1427] -> w1263 mode=indexing if=w1426
      i -> [w1427]
    }
    n456 = case shown="True" w1260 {
      tunnel: w1184 -> [w1279 w1292]
      tunnel: [w1280 w1291] -> w1259
      frame False {
        n457 = local read "SHIFT_DATA 2"() -> (w1282:string[])
        n458 = call "String To Time_4.vi"("error in (no error)"=w1279, "String Array In"=w1282) -> ("error out"=w1278:errorcluster, "Time Stamp Out"=w1277:timestamp[])  [unwired: 8 in]
        "Time Stamp Out 4" <- w1277
        n459 = Get Date/Time In Seconds() -> (seconds since 1Jan1904=w1281:timestamp)
        n460 = call "Shift Calculation_4.vi"("error in (no error)"=w1278, "Current Time"=w1281, "Time Stamp Out"=w1277) -> ("error out"=w1276:errorcluster, "Shift"=w1275:i32)  [unwired: 7 in]
        n461 = call <vilib>:"Clear Errors.vi"("error in (no error)"=w1276) -> ()  [unwired: 5 in, 2 out]
        n462 = case shown="4" w1275 {
          tunnel: ["A" "B" "C" "D"] -> w1280
          frame 1, Default {
          }
          frame 2 {
          }
          frame 3 {
          }
          frame 4 {
          }
        }
      }
      frame True {
        n463 = local read "SHIFT_DATA"() -> (w1290:string[])
        n464 = call "String To Time.vi"("error in (no error)"=w1292, "String Array In"=w1290) -> ("error out"=w1289:errorcluster, "Time Stamp Out"=w1294:timestamp[])  [unwired: 8 in]
        "Time Stamp Out" <- w1294
        n465 = Get Date/Time In Seconds() -> (seconds since 1Jan1904=w1293:timestamp)
        n466 = call "Shift Calculation.vi"("error in (no error)"=w1289, "Current Time"=w1293, "Time Stamp Out"=w1294) -> ("error out"=w1288:errorcluster, "Shift"=w1287:i32)  [unwired: 7 in]
        "Shift 4" <- w1287
        n467 = call <vilib>:"Clear Errors.vi"("error in (no error)"=w1288) -> ()  [unwired: 5 in, 2 out]
        n468 = case shown="3" w1287 {
          tunnel: ["A" "B" "C"] -> w1291
          frame 1, Default {
          }
          frame 2 {
          }
          frame 3 {
          }
        }
      }
    }
    "SHIFT" <- w1259
    n469 = for {
      tunnel: w1263 -> [w1298] mode=indexing
      shift-right: [w1302] -> w1256
      shift-left: w1262 -> [w1301]
      shift-right: [w1300] -> w1255
      shift-left: w1184 -> [w1299]
      n470 = case shown="1" w1298 {
        tunnel: [w1304 w1310 w1316 w1324 w1329 w1337 w1343 w1351 w1358 w1365 w1372 w1383 w1395 w1412 w1415 w1419 w1424] -> w1302
        tunnel: w1301 -> [w1306 w1312 w1318 w1326 w1331 w1339 w1345 w1353 w1360 w1367 w1373 w1384 w1396 w1412 w1415 w1416 w1421]
        tunnel: [w1303 w1309 w1315 w1323 w1328 w1336 w1342 w1350 w1357 w1364 w1371 w1382 w1394 w1411 w1414 w1418 w1423] -> w1300
        tunnel: w1299 -> [w1305 w1311 w1317 w1325 w1330 w1338 w1344 w1352 w1359 w1366 w1369 w1380 w1392 w1411 w1414 w1417 w1422]
        frame -1, Default {
          # "DEFAULT"
          n471 = Enqueue Element(queue=w1306, element=cluster{"CASE":T11} {"CASE"=enum."-1"}, error in (no error)=w1305) -> (queue out=w1304:refnum<queue>, error out=w1303:errorcluster)  [unwired: 1 in, 1 out]
        }
        frame 0 {
          # "SCAN BARCODE OP 10"
          n472 = Enqueue Element(queue=w1312, element=cluster{"CASE":T11} {"CASE"=enum."SCAN1"}, error in (no error)=w1311) -> (queue out=w1310:refnum<queue>, error out=w1309:errorcluster)  [unwired: 1 in, 1 out]
        }
        frame 1 {
          # "DATALOG OF ST 1"
          n473 = disable-structure shown="Enabled" {
            disable-tunnel: [w1319 w1320] -> w1313
            frame Enabled {
              n474 = local read "OP 10 & OP 21"() -> (w1319:T2)
            }
            frame Disabled {
              n475 = local read item#-1() -> (w1320)
            }
          }
          "STATION-1 2" <- w1313
          n476 = Enqueue Element(queue=w1318, element=cluster{"CASE":T11} {"CASE"=enum."DATALOG1"}, error in (no error)=w1317) -> (queue out=w1316:refnum<queue>, error out=w1315:errorcluster)  [unwired: 1 in, 1 out]
        }
        frame 2 {
          # "SCAN BARCODE FOR ST 2"
          n477 = global write "DATA LOG.vi" "op 30"(0 ("op 30")) -> ()
          n478 = Enqueue Element(queue=w1326, element=cluster{"CASE":T11} {"CASE"=enum."SCAN2"}, error in (no error)=w1325) -> (queue out=w1324:refnum<queue>, error out=w1323:errorcluster)  [unwired: 1 in, 1 out]
        }
        frame 3 {
          # "DATALOG OF ST 2"
          n479 = disable-structure shown="Enabled" {
            disable-tunnel: [w1332 w1333] -> _
            frame Disabled {
              n480 = local read item#-1() -> (w1332)
            }
            frame Enabled {
              n481 = local read item#-1() -> (w1333)
            }
          }
          n482 = Enqueue Element(queue=w1331, element=cluster{"CASE":T11} {"CASE"=enum."DATALOG2"}, error in (no error)=w1330) -> (queue out=w1329:refnum<queue>, error out=w1328:errorcluster)  [unwired: 1 in, 1 out]
        }
        frame 4 {
          # "SCAN BARCODE FOR ST 3"
          n483 = global write "DATA LOG.vi" "op 40"(0 ("op 30")) -> ()
          n484 = Enqueue Element(queue=w1339, element=cluster{"CASE":T11} {"CASE"=enum."SCAN3"}, error in (no error)=w1338) -> (queue out=w1337:refnum<queue>, error out=w1336:errorcluster)  [unwired: 1 in, 1 out]
        }
        frame 5 {
          # "DATALOG OF ST 3"
          n485 = disable-structure shown="Enabled" {
            disable-tunnel: [w1346 w1347] -> w1340
            frame Disabled {
              n486 = local read "OP 40"() -> (w1346:T6)
            }
            frame Enabled {
              n487 = local read "OP 40"() -> (w1347:T6)
            }
          }
          "STATION-3 2" <- w1340
          n488 = Enqueue Element(queue=w1345, element=cluster{"CASE":T11} {"CASE"=enum."DATALOG3"}, error in (no error)=w1344) -> (queue out=w1343:refnum<queue>, error out=w1342:errorcluster)  [unwired: 1 in, 1 out]
        }
        frame 6 {
          # "SCAN BARCODE FOR ST 4"
          n489 = global write "DATA LOG.vi" "op 60"(0 ("op 30")) -> ()
          n490 = Enqueue Element(queue=w1353, element=cluster{"CASE":T11} {"CASE"=enum."SCAN4"}, error in (no error)=w1352) -> (queue out=w1351:refnum<queue>, error out=w1350:errorcluster)  [unwired: 1 in, 1 out]
        }
        frame 7 {
          # "DATALOG OF ST 4"
          n491 = disable-structure shown="Enabled" {
            disable-tunnel: [w1361 w1362] -> w1355
            frame Enabled {
              n492 = local read "OP 61"() -> (w1361:T1)
            }
            frame Disabled {
              n493 = local read "OP 60"() -> (w1362:T7)
            }
          }
          "STATION-4 2" <- w1355
          n494 = Enqueue Element(queue=w1360, element=cluster{"CASE":T11} {"CASE"=enum."DATALOG4"}, error in (no error)=w1359) -> (queue out=w1358:refnum<queue>, error out=w1357:errorcluster)  [unwired: 1 in, 1 out]
          "DATA" <- TRUE
        }
        frame 8 {
          # "DATALOG OF ST 4"
          n495 = Enqueue Element(queue=w1367, element=cluster{"CASE":T11} {"CASE"=enum."-1"}, error in (no error)=w1366) -> (queue out=w1365:refnum<queue>, error out=w1364:errorcluster)  [unwired: 1 in, 1 out]
        }
        frame 9 {
          # "FOR ST 2 : ON CYCLE START BIT WRITE BARCODE STATUS '0' TO PLC"
          n496 = flat-sequence {
            tunnel: [w1375] -> w1368
            tunnel: w1369 -> [w1376]
            frame #0 {
              n497 = global write "DATA LOG.vi" "OP30 ST 2 STRING"("" ("OP30 ST 2 STRING")) -> ()
              n498 = call "PADMINI_AUTO_BARCODE_STATUS2.vi"("Enum"=enum16{"Read", "Write"}."Write", "error in (no error)"=w1376, "I/P"=u16 0) -> ("error out"=w1375:errorcluster)  [unwired: 7 in, 1 out]
            }
          }
          n499 = Enqueue Element(queue=w1373, element=cluster{"CASE":T11} {"CASE"=enum."-1"}, error in (no error)=w1368) -> (queue out=w1372:refnum<queue>, error out=w1371:errorcluster)  [unwired: 1 in, 1 out]
        }
        frame 10 {
          # "FOR ST 3 : ON CYCLE START BIT WRITE BARCODE STATUS '0' TO PLC"
          n500 = flat-sequence {
            tunnel: [w1389] -> w1379
            tunnel: w1380 -> [w1390]
            frame #0 {
              n501 = global write "DATA LOG.vi" "ST 3 STRING 2"("" ("OP30 ST 2 STRING")) -> ()
              n502 = global write "DATA LOG.vi" "scan op 40"(TRUE ("scan op 40")) -> ()
              n503 = call "PADMINI_AUTO_BARCODE_STATUS3.vi"("Enum"=enum16{"Read", "Write"}."Write", "error in (no error)"=w1390, "I/P"=u16 0) -> ("error out"=w1389:errorcluster)  [unwired: 7 in, 1 out]
            }
          }
          n504 = Enqueue Element(queue=w1384, element=cluster{"CASE":T11} {"CASE"=enum."-1"}, error in (no error)=w1379) -> (queue out=w1383:refnum<queue>, error out=w1382:errorcluster)  [unwired: 1 in, 1 out]
        }
        frame 11 {
          # "FOR ST 4 : ON CYCLE START BIT WRITE BARCODE STATUS '0' TO PLC"
          n505 = flat-sequence {
            tunnel: w1392 -> [w1398]
            tunnel: [w1397] -> w1391
            frame #0 {
              n506 = disable-structure shown="Enabled" {
                disable-tunnel: w1398 -> [w1402 w1406]
                disable-tunnel: [w1400 w1408] -> w1397
                frame Disabled {
                  n507 = global write "DATA LOG.vi" "scan op 60"(TRUE ("scan op 60")) -> ()
                  n508 = global write "DATA LOG.vi" "ST 4 STRING 3"("") -> ()
                  n509 = call "PADMINI_AUTO_BARCODE_STATUS4.vi"("Enum"=enum16{"Read", "Write"}."Write", "error in (no error)"=w1402, "I/P"=u16 0) -> ("error out"=w1400:errorcluster)  [unwired: 7 in, 1 out]
                }
                frame Enabled {
                  n510 = call <vilib>:"Clear Errors.vi"("error in (no error)"=w1406) -> ("error out"=w1405:errorcluster)  [unwired: 5 in, 1 out]
                  n511 = call "PADMINI_AUTO_BARCODE_STATUS4.vi"("Enum"=enum16{"Read", "Write"}."Write", "error in (no error)"=w1405, "I/P"=u16 0) -> ("error out"=w1408:errorcluster)  [unwired: 7 in, 1 out]
                }
              }
            }
          }
          n512 = Enqueue Element(queue=w1396, element=cluster{"CASE":T11} {"CASE"=enum."-1"}, error in (no error)=w1391) -> (queue out=w1395:refnum<queue>, error out=w1394:errorcluster)  [unwired: 1 in, 1 out]
        }
        frame 12 {
          n513 = property on="Tab Control" class="TabCtl (strict)"("Value"=enum32{"Page 1", "Page 2"}."Page 2" ("Tab Control")) -> ()  [unwired: 2 in, 2 out]
        }
        frame 13 {
          n514 = property on="Tab Control" class="TabCtl (strict)"("Value"=enum32{"Page 1", "Page 2"}."Page 1" ("Tab Control")) -> ()  [unwired: 2 in, 2 out]
        }
        frame 14 {
          n515 = Enqueue Element(queue=w1416, element=cluster{"CASE":T11} {"CASE"=enum."BARCODE RECIPE"}, error in (no error)=w1417) -> (queue out=w1419:refnum<queue>, error out=w1418:errorcluster)  [unwired: 1 in, 1 out]
        }
        frame 15 {
          n516 = Enqueue Element(queue=w1421, element=cluster{"CASE":T11} {"CASE"=enum."EMERGENCY STOP"}, error in (no error)=w1422) -> (queue out=w1424:refnum<queue>, error out=w1423:errorcluster)  [unwired: 1 in, 1 out]
        }
      }
    }
    n517 = case shown="False" "stop 2" {
      tunnel: w1256 -> [w1266 w1272]
      tunnel: [w1266 w1271] -> w1254
      tunnel: w1255 -> [w1265 w1270]
      tunnel: [w1265 w1269] -> w1253
      tunnel: [FALSE TRUE] -> w1252
      frame False {
      }
      frame True {
        n518 = Flush Queue(queue=w1272, error in (no error)=w1270) -> (queue out=w1274:refnum<queue>, error out=w1273:errorcluster)  [unwired: 1 out]
        n519 = Enqueue Element(queue=w1274, element=cluster{"CASE":T11} {"CASE"=enum."STOP"}, error in (no error)=w1273) -> (queue out=w1271:refnum<queue>, error out=w1269:errorcluster)  [unwired: 1 in, 1 out]
      }
    }
    "stop" <- w1252
    n520 = Wait (ms)(milliseconds to wait=u32 50) -> ()  [unwired: 1 out]
  }
  n521 = while {
    tunnel: w19 -> [w1444]
    tunnel: w41 -> [w1443]
    tunnel: w39 -> [w1441]
    tunnel: w40 -> [w1440]
    tunnel: w42 -> [w1439]
    tunnel: [w1429] -> w44
    stop <- w1438 stop-if-true
    # "Output Indicator"
    n522 = flat-sequence {
      tunnel: w1444 -> [w1467]
      tunnel: w1443 -> [w1511]
      tunnel: [w1453] -> w1442
      tunnel: w1441 -> [w1507]
      tunnel: w1440 -> [w1506]
      tunnel: w1439 -> [w1505]
      tunnel: [w1507] -> w1436
      tunnel: [w1506] -> w1434
      tunnel: [w1505] -> w1430
      tunnel: w1442 -> [w1547]
      tunnel: [w1543] -> w1437
      tunnel: w1436 -> [w1563]
      tunnel: [w1562] -> w1435
      tunnel: w1434 -> [w1562]
      tunnel: [w1561] -> w1431
      tunnel: w1430 -> [w1561]
      tunnel: w1437 -> [w1586]
      tunnel: w1435 -> [w1621]
      tunnel: [w1620] -> w1433
      tunnel: [w1619] -> w1432
      tunnel: w1431 -> [w1619]
      tunnel: w1433 -> [w1640]
      tunnel: [w1715] -> w1429
      tunnel: w1432 -> [w1714]
      frame #0 {
        w1489 = 1.0 ("element")
        # "CYCLE STATUS"
        n523 = call "PADMINI_AUTO_BARCODE_STRING.vi"("Enum"=enum16{"Read", "Write"}."Read", "error in (no error)"=w1467) -> ("Input 2"=w1513:string)  [unwired: 8 in, 1 out]
        n524 = call "PADMINI_AUTO_COUNTER_TIME.vi"("Enum"=enum16{"Read", "Write"}."Read", "error in (no error)"=w1467) -> ("Input 2"=w1517:u16[])  [unwired: 8 in, 1 out]
        n525 = call "PADMINI_AUTO_CYCLE_BIT.vi"("Enum"=enum16{"Read", "Write"}."Read", "error in (no error)"=w1467) -> ("Input 2"=w1509:u16[])  [unwired: 8 in, 1 out]
        n526 = property on="OP 10 & OP 21" class="Clust"(error in=w1467) -> (error out=w1452:errorcluster, "Controls[]"=w1466:refnum<vi>[])  [unwired: 1 in, 1 out]
        n527 = call "PADMINI_AUTO_RESULT_DATA.vi"("Enum"=enum16{"Read", "Write"}."Read", "error in (no error)"=w1467) -> ("Input 2"=w1447:dbl[])  [unwired: 8 in, 1 out]
        n528 = call "PADMINI_AUTO_RESULT_DATA_st1_log.vi"("Enum"=enum16{"Read", "Write"}."Read", "error in (no error)"=w1467) -> ("Input 2"=w1482:dbl[])  [unwired: 8 in, 1 out]
        n529 = Index Array(array=w1517) -> (element #1=w1488:u16, element #2=w1516:u16, element #3=w1515:u16, element #4=w1514:u16)  [unwired: 4 in]
        n530 = Index Array(array=w1509) -> (element=w1508:u16)  [unwired: 1 in]
        n531 = Index Array(array=w1447) -> (element #1=w1450:dbl, element #2=w1451:dbl, element #3=w1504:dbl, element #4=w1503:dbl, element #5=w1502:dbl, element #6=w1501:dbl, element #7=w1500:dbl, element #8=w1499:dbl, element #9=w1498:dbl, element #10=w1497:dbl, element #11=w1496:dbl, element #12=w1495:dbl, element #13=w1494:dbl, element #14=w1493:dbl, element #15=w1492:dbl, element #16=w1491:dbl, element #17=w1490:dbl)  [unwired: 17 in]
        n532 = Index Array(array=w1482) -> (element #1=w1480:dbl, element #2=w1479:dbl, element #3=w1478:dbl, element #4=w1477:dbl, element #5=w1476:dbl, element #6=w1475:dbl, element #7=w1474:dbl, element #8=w1473:dbl, element #9=w1472:dbl, element #10=w1471:dbl, element #11=w1470:dbl, element #12=w1469:dbl, element #13=w1468:dbl, element #16=w1455:dbl)  [unwired: 16 in, 2 out]
        n533 = Index Array(array=w1511, index=w1508) -> (element=w1448:string)
        n534 = Array Subset(array=w1447, index=15, length=10) -> (w1459:dbl[])
        n535 = Array Subset(array=w1466, index=15, length=8) -> (w1463:refnum<vi>[])
        n536 = for {
          shift-right: [w1532] -> w1449
          shift-left: w1452 -> [w1532]
          tunnel: w1463 -> [w1534] mode=indexing
          tunnel: [w1531] -> w1462 mode=indexing
          w1533 = refnum<vi> refnum  # Boolean
          n537 = To More Specific Class(target class=w1533, reference=w1534) -> (specific class reference=w1531:refnum<vi>)  [unwired: 1 in, 1 out]
        }
        n538 = for {
          shift-right: [w1539] -> w1484
          shift-left: _ -> [w1539]
          tunnel: w1459 -> [_] mode=indexing
          tunnel: [w1538] -> w1526 mode=indexing
          w1540 = refnum<vi> refnum  # Boolean
          n539 = To More Specific Class(target class=w1540) -> (specific class reference=w1538:refnum<vi>)  [unwired: 2 in, 1 out]
        }
        n540 = Divide(x=w1488, y=10.0) -> (x/y=w1487:dbl)
        n541 = Build Array(w1496, w1495, w1494, w1493, w1492, w1491, w1490, w1489, w1489, w1489) -> (w1522:dbl[])
        n542 = Build Array(w1474, w1473, w1472, w1471, w1470, w1469, w1468) -> (w1460:dbl[])
        n543 = Bundle By Name("STATUS"=w1448, "BARCODE"=w1513, "Cycle Time"=w1487, "OK Part"=w1516, "NOK Part"=w1515, "Total"=w1514, "Load at 13.4 mm(N)"=w1450, "Load at 14 mm(N)"=w1451, "Seal Press Load (N)"=w1504, "Spring Height (mm)"=w1503, "Spring and Seal Press Load(N)"=w1502, "Spring & Seal Press Check Load(N)"=w1501, "PARAMETER 7"=w1500, "PARAMETR 8"=w1499, "PARAMETER 9"=w1498, "PARAMETER 10"=w1497) -> ()  [unwired: 1 in, 1 out]
        n544 = for {
          tunnel: w1526 -> [w1537] mode=indexing
          tunnel: w1522 -> [w1536] mode=indexing
          tunnel: w1484 -> [_]
          tunnel: [w1535] -> w1454
          n545 = call "PADMINI_BOOL_COLOR_CHANGE.vi"("Numeric"=w1536, "Boolean in"=w1537) -> ("error out"=w1535:errorcluster)  [unwired: 9 in]
        }
        n546 = for {
          tunnel: w1462 -> [w1530] mode=indexing
          tunnel: w1460 -> [w1529] mode=indexing
          tunnel: w1449 -> [w1528]
          tunnel: [w1527] -> w1458
          n547 = call "PADMINI_BOOL_COLOR_CHANGE.vi"("error in (no error)"=w1528, "Numeric"=w1529, "Boolean in"=w1530) -> ("error out"=w1527:errorcluster)  [unwired: 8 in]
        }
        "error out" <- w1458
        n548 = control-ref of="CYCLE RESULT"() -> (w1456:refnum<vi>)
        n549 = local read item#-1() -> ()  [unwired: 1 out]
        n550 = local read "OP 10 & OP 21"() -> (w1461:T2)
        n551 = Bundle By Name(cluster=w1461, "SPRING LOAD AT 13.4 mm(N)"=w1480, "SPRING LOAD AT 14 mm((N)"=w1479, "SEAL PRESS LOAD(N)"=w1478, "SPRING HEIGHT(mm)"=w1477, "SPRING AND SEAL PRESS LOAD(N)"=w1476, "SPRING AND SEAL PRESS CHECK LOAD(N)"=w1475) -> (→"OP 10 & OP 21":T2)
        n552 = call "PADMINI_AUTO_CYCLE STATE.vi"("Enum"=enum16{"Read", "Write"}."Read", "error in (no error)"=w1454) -> ("error out"=w1453:errorcluster, "Input 2"=w1520:u16[])  [unwired: 8 in]
        n553 = call "PADMINI_RESULT_COLOR_CHANGE .vi"("Numeric"=w1455, "Boolean in"=w1456) -> ()  [unwired: 10 in]
        n554 = Index Array(array=w1520, index #1=0 ("index")) -> (element #1=w1485:u16, element #3=w1457:u16)  [unwired: 2 in, 1 out]
        n555 = call "PADMINI_STATUS_COLOR_CHANGE .vi"("Numeric"=w1485) -> ()  [unwired: 11 in]
        n556 = call "PADMINI_RESULT_COLOR_CHANGE .vi"("Numeric"=w1457) -> ()  [unwired: 11 in]
      }
      frame #1 {
        n557 = call "PADMINI_AUTO_CYCLE_BIT2.vi"("Enum"=enum16{"Read", "Write"}."Read", "error in (no error)"=w1547) -> ("Input 2"=w1577:u16[])  [unwired: 8 in, 1 out]
        n558 = call "PADMINI_AUTO_BARCODE_STRING2.vi"("Enum"=enum16{"Read", "Write"}."Read", "error in (no error)"=w1547) -> ()  [unwired: 8 in, 2 out]
        n559 = call "PADMINI_AUTO_COUNTER_TIME2.vi"("Enum"=enum16{"Read", "Write"}."Read", "error in (no error)"=w1547) -> ("Input 2"=w1570:u16[])  [unwired: 8 in, 1 out]
        n560 = call "PADMINI_AUTO_RESULT_DATA2.vi"("Enum"=enum16{"Read", "Write"}."Read", "error in (no error)"=w1547) -> ("Input 2"=w1565:dbl[])  [unwired: 8 in, 1 out]
        n561 = Index Array(array=w1570) -> (element #1=w1571:u16, element #2=w1572:u16, element #3=w1573:u16, element #4=w1574:u16)  [unwired: 4 in]
        n562 = Index Array(array=w1577) -> (element=w1578:u16)  [unwired: 1 in]
        n563 = Index Array(array=w1565) -> (element #1=w1560:dbl, element #2=w1559:dbl, element #3=w1558:dbl, element #4=w1557:dbl, element #5=w1556:dbl, element #6=w1555:dbl, element #7=w1554:dbl, element #8=w1553:dbl, element #9=w1552:dbl, element #10=w1551:dbl, element #11=w1550:dbl, element #12=w1549:dbl)  [unwired: 12 in]
        n564 = Index Array(array=w1563, index=w1578) -> (element=w1579:string)
        n565 = call "PADMINI_BOOL_COLOR_CHANGE.vi"("error in (no error)"=w1547, "Numeric"=w1550) -> ("error out"=w1548:errorcluster)  [unwired: 9 in]
        n566 = Divide(x=w1571, y=u16 10) -> (x/y=w1542:dbl)
        n567 = call "PADMINI_BOOL_COLOR_CHANGE.vi"("error in (no error)"=w1548, "Numeric"=w1549) -> ("error out"=w1545:errorcluster)  [unwired: 9 in]
        n568 = call "PADMINI_AUTO_CYCLE STATE2.vi"("Enum"=enum16{"Read", "Write"}."Read", "error in (no error)"=w1545) -> ("error out"=w1543:errorcluster, "Input 2"=w1567:u16[])  [unwired: 8 in]
        n569 = local read item#-1() -> ()  [unwired: 1 out]
        n570 = Bundle By Name("STATUS"=w1579, "Cycle Time"=w1542, "OK Part"=w1572, "NOK Part"=w1573, "Total"=w1574, "Force (KgF)"=w1560, "POSITION (mm)"=w1559, "PARAMETER 3"=w1558, "PARAMETER 4"=w1557, "PARAMETER 5"=w1556, "PARAMETER 6"=w1555, "PARAMETER 7"=w1554, "PARAMETER 8"=w1553, "PARAMETER 9"=w1552, "PARAMETER 10"=w1551) -> ()  [unwired: 1 in, 1 out]
        n571 = Index Array(array=w1567, index #1=0 ("index")) -> (element #1=w1546:u16, element #3=w1544:u16)  [unwired: 2 in, 1 out]
        n572 = call "PADMINI_RESULT_COLOR_CHANGE .vi"("Numeric"=w1544) -> ()  [unwired: 11 in]
        n573 = call "PADMINI_STATUS_COLOR_CHANGE .vi"("Numeric"=w1546) -> ()  [unwired: 11 in]
      }
      frame #2 {
        n574 = call "PADMINI_AUTO_RESULT_DATA3.vi"("Enum"=enum16{"Read", "Write"}."Read", "error in (no error)"=w1586) -> ("Input 2"=w1636:dbl[])  [unwired: 8 in, 1 out]
        n575 = Index Array(array=w1636) -> (element #1=w1618:dbl, element #2=w1617:dbl, element #3=w1583:dbl, element #4=w1616:dbl, element #5=w1615:dbl, element #6=w1614:dbl, element #7=w1613:dbl, element #8=w1612:dbl, element #9=w1611:dbl, element #10=w1610:dbl, element #11=w1598:dbl, element #12=w1597:dbl, element #13=w1596:dbl, element #14=w1595:dbl, element #15=w1594:dbl, element #16=w1593:dbl, element #17=w1592:dbl)  [unwired: 20 in, 3 out]
        n576 = control-ref of="FLUSHING FLOW RATE"() -> (w1605:refnum<vi>)
        n577 = call "PADMINI_AUTO_CYCLE_BIT3.vi"("Enum"=enum16{"Read", "Write"}."Read", "error in (no error)"=w1586) -> ("Input 2"=w1624:u16[])  [unwired: 8 in, 1 out]
        n578 = call "PADMINI_AUTO_BARCODE_STRING3.vi"("Enum"=enum16{"Read", "Write"}."Read", "error in (no error)"=w1586) -> ()  [unwired: 8 in, 2 out]
        n579 = call "PADMINI_AUTO_COUNTER_TIME3.vi"("Enum"=enum16{"Read", "Write"}."Read", "error in (no error)"=w1586) -> ("Input 2"=w1630:u16[])  [unwired: 8 in, 1 out]
        n580 = control-ref of="FLUSHING PRESSURE"() -> (w1604:refnum<vi>)
        n581 = call "PADMINI_BOOL_COLOR_CHANGE.vi"("error in (no error)"=w1586, "Numeric"=w1598, "Boolean in"=w1605) -> ("error out"=w1591:errorcluster)  [unwired: 8 in]
        n582 = Index Array(array=w1630) -> (element #1=w1607:u16, element #2=w1629:u16, element #3=w1628:u16, element #4=w1627:u16)  [unwired: 4 in]
        n583 = Index Array(array=w1624) -> (element=w1623:u16)  [unwired: 1 in]
        n584 = control-ref of="CALIBRATION LOAD VALUE"() -> (w1603:refnum<vi>)
        n585 = control-ref of="CALIBRATION DISPLACEMENT VALUE"() -> (w1602:refnum<vi>)
        n586 = control-ref of="CALIBRATION FLOW RATE"() -> (w1601:refnum<vi>)
        n587 = control-ref of="CALIBRATION PRESSURE"() -> (w1600:refnum<vi>)
        n588 = control-ref of="FIXING RING DISPLACEMENT"() -> (w1599:refnum<vi>)
        n589 = call "PADMINI_BOOL_COLOR_CHANGE.vi"("error in (no error)"=w1591, "Numeric"=w1597, "Boolean in"=w1604) -> ("error out"=w1590:errorcluster)  [unwired: 8 in]
        n590 = Divide(x=w1607, y=10.0) -> (x/y=w1606:dbl)
        n591 = Index Array(array=w1621, index=w1623) -> (element=w1622:string)
        n592 = call "PADMINI_BOOL_COLOR_CHANGE.vi"("error in (no error)"=w1590, "Numeric"=w1596, "Boolean in"=w1603) -> ("error out"=w1589:errorcluster)  [unwired: 8 in]
        n593 = call "PADMINI_BOOL_COLOR_CHANGE.vi"("error in (no error)"=w1589, "Numeric"=w1595, "Boolean in"=w1602) -> ("error out"=w1588:errorcluster)  [unwired: 8 in]
        n594 = call "PADMINI_BOOL_COLOR_CHANGE.vi"("error in (no error)"=w1588, "Numeric"=w1594, "Boolean in"=w1601) -> ("error out"=w1587:errorcluster)  [unwired: 8 in]
        n595 = call "PADMINI_BOOL_COLOR_CHANGE.vi"("error in (no error)"=w1587, "Numeric"=w1593, "Boolean in"=w1600) -> ("error out"=w1585:errorcluster)  [unwired: 8 in]
        n596 = call "PADMINI_BOOL_COLOR_CHANGE.vi"("error in (no error)"=w1585, "Numeric"=w1592, "Boolean in"=w1599) -> ("error out"=w1584:errorcluster)  [unwired: 8 in]
        n597 = local read "OP 40"() -> (w1638:T6)
        n598 = Bundle By Name(cluster=w1638, "STATUS"=w1622, "Cycle Time"=w1606, "OK Part"=w1629, "NOK Part"=w1628, "Total"=w1627, "Flushing Flow (Lph)"=w1618, "Flushing Pressure (Bar)"=w1617, "Calibration Load (KgF)"=w1583, "Calibration Displacement (mm)"=w1616, "Calibration Flow Rate (Lph)"=w1615, "Calibration Pressure (Bar)"=w1614, "Fixing Ring Displacement (mm)"=w1613, "PARAMETER 8"=w1612, "PARAMETER 9"=w1611, "PARAMETER 10"=w1610) -> (→"OP 40":T6)
        n599 = call "PADMINI_AUTO_CYCLE STATE3.vi"("Enum"=enum16{"Read", "Write"}."Read", "error in (no error)"=w1584) -> ("error out"=w1620:errorcluster, "Input 2"=w1634:u16[])  [unwired: 8 in]
        n600 = control-ref of="Cycle Status"() -> (w1580:refnum<vi>)
        n601 = control-ref of="Cycle Result"() -> (w1581:refnum<vi>)
        n602 = Index Array(array=w1634, index #1=0 ("index")) -> (element #1=w1633:u16, element #3=w1582:u16)  [unwired: 2 in, 1 out]
        n603 = call "PADMINI_STATUS_COLOR_CHANGE .vi"("Numeric"=w1633, "Boolean in"=w1580) -> ()  [unwired: 10 in]
        n604 = call "PADMINI_RESULT_COLOR_CHANGE .vi"("Numeric"=w1582, "Boolean in"=w1581) -> ()  [unwired: 10 in]
      }
      frame #3 {
        w1679 = 1.0 ("element")
        n605 = property on="OP 61" class="Clust"(error in=w1640) -> (error out=w1665:errorcluster, "Controls[]"=w1663:refnum<vi>[])  [unwired: 1 in, 1 out]
        n606 = property on="OP 60" class="Clust"(error in=w1640) -> (error out=w1672:errorcluster, "Controls[]"=w1690:refnum<vi>[])  [unwired: 1 in, 1 out]
        n607 = call "PADMINI_AUTO_CYCLE_BIT4.vi"("Enum"=enum16{"Read", "Write"}."Read", "error in (no error)"=w1640) -> ("Input 2"=w1711:u16[])  [unwired: 8 in, 1 out]
        n608 = call "PADMINI_AUTO_BARCODE_STRING4.vi"("Enum"=enum16{"Read", "Write"}."Read", "error in (no error)"=w1640) -> ()  [unwired: 8 in, 2 out]
        n609 = call "PADMINI_AUTO_COUNTER_TIME4.vi"("Enum"=enum16{"Read", "Write"}."Read", "error in (no error)"=w1640) -> ("Input 2"=w1704:u16[])  [unwired: 8 in, 1 out]
        n610 = call <vilib>:"Clear Errors.vi"("error in (no error)"=w1640) -> ("error out"=w1639:errorcluster)  [unwired: 5 in, 1 out]
        n611 = call "PADMINI_AUTO_RESULT_DATA_st4_log.vi"("Enum"=enum16{"Read", "Write"}."Read", "error in (no error)"=w1639) -> ("Input 2"=w1657:dbl[])  [unwired: 8 in, 1 out]
        n612 = call "PADMINI_AUTO_RESULT_DATA4.vi"("Enum"=enum16{"Read", "Write"}."Read", "error in (no error)"=w1640) -> ("Input 2"=w1696:dbl[])  [unwired: 8 in, 1 out]
        n613 = Index Array(array=w1704) -> (element #1=w1705:u16, element #2=w1706:u16, element #3=w1707:u16, element #4=w1708:u16)  [unwired: 4 in]
        n614 = Index Array(array=w1711) -> (element=w1712:u16)  [unwired: 1 in]
        n615 = Index Array(array=w1696) -> (element #1=w1697:dbl, element #2=w1678:dbl, element #3=w1688:dbl, element #4=w1677:dbl, element #5=w1687:dbl, element #6=w1686:dbl, element #7=w1685:dbl, element #8=w1684:dbl, element #9=w1683:dbl, element #10=w1682:dbl, element #11=w1646:dbl, element #12=w1681:dbl, element #13=w1680:dbl)  [unwired: 13 in]
        n616 = Array Subset(array=w1663, index=15, length=3) -> (w1662:refnum<vi>[])
        n617 = Index Array(array=w1657) -> (element #1=w1656:dbl, element #2=w1655:dbl, element #3=w1654:dbl, element #4=w1653:dbl, element #5=w1652:dbl, element #6=w1651:dbl, element #7=w1650:dbl)  [unwired: 8 in, 1 out]
        n618 = Array Subset(array=w1690, index=15, length=10) -> (w1691:refnum<vi>[])
        n619 = Index Array(array=w1714, index=w1712) -> (element=w1713:string)
        n620 = for {
          shift-right: [w1729] -> w1666
          shift-left: w1665 -> [w1729]
          tunnel: w1662 -> [w1731] mode=indexing
          tunnel: [w1728] -> w1664 mode=indexing
          w1730 = refnum<vi> refnum  # Boolean
          n621 = To More Specific Class(target class=w1730, reference=w1731) -> (specific class reference=w1728:refnum<vi>)  [unwired: 1 in, 1 out]
        }
        n622 = for {
          shift-right: [w1737] -> w1671
          shift-left: w1672 -> [w1737]
          tunnel: w1691 -> [w1739] mode=indexing
          tunnel: [w1736] -> w1674 mode=indexing
          w1738 = refnum<vi> refnum  # Boolean
          n623 = To More Specific Class(target class=w1738, reference=w1739) -> (specific class reference=w1736:refnum<vi>)  [unwired: 1 in, 1 out]
        }
        n624 = Build Array(w1652, w1651, w1650) -> (w1649:dbl[])
        n625 = Divide(x=w1705, y=u16 10) -> (x/y=w1648:dbl)
        n626 = local read "OP 61"() -> (w1668:T1)
        n627 = Build Array(w1646, w1681, w1680, w1679, w1679, w1679, w1679, w1679, w1679, w1679) -> (w1698:dbl[])
        n628 = for {
          tunnel: w1664 -> [w1727] mode=indexing
          tunnel: w1649 -> [w1726] mode=indexing
          tunnel: w1666 -> [w1725]
          tunnel: [w1724] -> w1667
          n629 = call "PADMINI_BOOL_COLOR_CHANGE.vi"("error in (no error)"=w1725, "Numeric"=w1726, "Boolean in"=w1727) -> ("error out"=w1724:errorcluster)  [unwired: 8 in]
        }
        n630 = for {
          tunnel: w1674 -> [w1735] mode=indexing
          tunnel: w1698 -> [w1734] mode=indexing
          tunnel: w1671 -> [w1733]
          tunnel: [w1732] -> w1670
          n631 = call "PADMINI_BOOL_COLOR_CHANGE.vi"("error in (no error)"=w1733, "Numeric"=w1734, "Boolean in"=w1735) -> ("error out"=w1732:errorcluster)  [unwired: 8 in]
        }
        n632 = Equal?(x=w1646, y=1.0) -> (x = y?=w1644:bool)
        n633 = disable-structure shown="Enabled" {
          disable-tunnel: w1667 -> [w1722 w1723]
          disable-tunnel: [w1716 w1723] -> w1659
          frame Disabled {
            n634 = call "PADMINI_AUTO_CYCLE STATE4.vi"("Enum"=enum16{"Read", "Write"}."Read", "error in (no error)"=w1722) -> ("error out"=w1716:errorcluster, "Input 2"=w1720:u16[])  [unwired: 8 in]
            n635 = control-ref of="Cycle Result"() -> (w1718:refnum<vi>)
            n636 = Index Array(array=w1720, index #1=0 ("index")) -> (element #3=w1717:u16)  [unwired: 2 in, 2 out]
            n637 = call "PADMINI_RESULT_COLOR_CHANGE .vi"("Numeric"=w1717, "Boolean in"=w1718) -> ()  [unwired: 10 in]
          }
          frame Enabled {
          }
        }
        "error out 3" <- w1659
        n638 = Select(t=TRUE, s=w1644, f=FALSE) -> (s? t:f=w1641:bool)
        n639 = Bundle By Name(cluster=w1668, "Pressure (Bar)"=w1656, "Actual Flow (Lpm)"=w1655, "lt Pressure (Bar)"=w1654, "Actual Flow (ccm)"=w1653) -> (→"OP 61":T1)
        n640 = call "PADMINI_AUTO_CYCLE STATE4.vi"("Enum"=enum16{"Read", "Write"}."Read", "error in (no error)"=w1670) -> ("error out"=w1715:errorcluster, "Input 2"=w1700:u16[])  [unwired: 8 in]
        n641 = global write "Global 1.vi" "STATION 2 OK"(w1641) -> ()
        n642 = local read "OP 60"() -> (w1692:T7)
        n643 = Bundle By Name(cluster=w1692, "STATUS"=w1713, "Cycle Time"=w1648, "OK Part"=w1706, "NOK Part"=w1707, "Total"=w1708, "Actual Flow (Lpm)"=w1697, "Pressure (Bar)"=w1678, "Actual Flow (ccm)"=w1688, "Pressure (Bar)"=w1677, "PARAMETER 5"=w1687, "PARAMETER 6"=w1686, "PARAMETER 7"=w1685, "PARAMETER 8"=w1684, "PARAMETER 9"=w1683, "PARAMETER 10"=w1682) -> (→"OP 60":T7)
        n644 = control-ref of="Cycle Status"() -> (w1673:refnum<vi>)
        n645 = control-ref of="Cycle Result"() -> (w1675:refnum<vi>)
        n646 = Index Array(array=w1700, index #1=0 ("index")) -> (element #1=w1701:u16, element #3=w1676:u16)  [unwired: 2 in, 1 out]
        n647 = call "PADMINI_STATUS_COLOR_CHANGE .vi"("Numeric"=w1701, "Boolean in"=w1673) -> ()  [unwired: 10 in]
        n648 = call "PADMINI_RESULT_COLOR_CHANGE .vi"("Numeric"=w1676, "Boolean in"=w1675) -> ()  [unwired: 10 in]
      }
    }
    n649 = local read "stop"() -> (w1438:bool)
    n650 = disable-structure shown="Enabled" {
      disable-tunnel: [u32 1000 ("milliseconds to wait") u32 100 ("milliseconds to wait")] -> w1428
      frame Disabled {
      }
      frame Enabled {
      }
    }
    n651 = Wait (ms)(milliseconds to wait=w1428) -> ()  [unwired: 1 out]
  }
  n652 = Release Queue(queue=w96, error in (no error)=w102) -> (error out=w75:errorcluster)  [unwired: 1 in, 2 out]
  n653 = call <vilib>:"Clear Errors.vi"("error in (no error)"=w98) -> ("error out"=w79:errorcluster)  [unwired: 5 in, 1 out]
  n654 = call <vilib>:"DB Tools Close Connection.vi"("error in (no error)"=w79, "connection reference"=w97) -> ("error out"=w76:errorcluster)  [unwired: 5 in]
  n655 = Merge Errors(w75, w76, w44) -> (w77:errorcluster)
  n656 = call <vilib>:"Simple Error Handler.vi"("error in (no error)"=w77) -> ("error out"=w72:errorcluster)  [unwired: 4 in, 4 out]
  n657 = call <vilib>:"Clear Errors.vi"("error in (no error)"=w72) -> ("error out"=w78:errorcluster)  [unwired: 5 in, 1 out]
  n658 = flat-sequence {
    tunnel: w78 -> [w1741]
    tunnel: [w1741] -> w80
    frame #0 {
      n659 = global write "Global 1.vi" "REMOVE VI"(TRUE ("remove_VI")) -> ()
    }
  }
  n660 = property class="App"(error in=w80) -> (error out=w82:errorcluster, "App.Kind"=w81:T12)  [unwired: 1 in, 1 out]
  n661 = case shown="\"Development System\", Default" w81 {
    tunnel: [w1742 w1744] -> w83
    tunnel: w82 -> [w1742 w1743]
    frame "Development System", Default {
    }
    frame "Run Time System" {
      n662 = invoke class="VI" method="FP.Close"(error in=w1743) -> (error out=w1744:errorcluster)  [unwired: 2 in, 2 out]
    }
  }
  "error out 2" <- w83
